vi "Interfaz grafica - corriente.vi"() -> ()   [LabVIEW 2024]
uses:
  160620 Optotune Lens Driver 4 Labview package/Hello Optotune Lens (30.06.2015)/Calibration.ctl
  <vilib>/DAQmx/read.llb/DAQmx Read (Analog 1D Wfm NChan NSamp).vi
  <vilib>/Analysis/2dsp.llb/Decimate (single shot, DBL).vi
  <vilib>/Utility/file.llb/Read Delimited Spreadsheet (string).vi
  <vilib>/Instr/_visa.llb/VISA Configure Serial Port (Instr).vi
  <vilib>/DAQmx/create/channels.llb/DAQmx Create Channel (AI-Voltage-Basic).vi
  <vilib>/DAQmx/configure/timing.llb/DAQmx Timing (Sample Clock).vi
  <vilib>/DAQmx/miscellaneous.llb/DAQmx Fill In Error Info.vi
  <vilib>/Waveform/WDTOps.llb/WDT Index Channel DBL.vi
  <vilib>/Analysis/2dsp.llb/Decimate (continuous, DBL).vi
  <vilib>/Utility/file.llb/Write Delimited Spreadsheet (string).vi
  <vilib>/Waveform/WDTOps.llb/WDT Get Waveform Time Array DBL.vi
  <vilib>/Analysis/NI_AALPro.lvlib
panel:
  out "Array 4":string[](array[string])
  out "Array 3":string[](array[string])
  out "Array 2":string[](array[string])
  out "Array":string[](array[string])
  out "Nombre 2":string
  in  "Restablecer Iniciales":bool
  in  "Incremento":dbl=0.1 format="%#_13g"
  out "Potencia derecho":dbl
  out "error out 4":errorcluster
  out "error out 3":errorcluster
  out "error out 2":errorcluster
  in  "Tab Control 3":enum32{"WL", "Video"}(tab)
  out "Waveform length":dbl[][](graph)
  in  "Minimo escala Y":dbl format="%#_13g"
  in  "Maximo escala Y":dbl format="%#_13g"
  in  "Escala autom. Y":u8=1
  in  "Escala autom. X":u8=1
  in  "Maximo escala X":dbl
  in  "Minimo escala X":dbl
  out "VISA resource name out":string
  in  "Tab Control 2":T1(tab)
  in  "DAQmx Physical Channel":tag
  in  "Frecuencia muestreo":i32=20000
  in  "tamaño buffer":i32=1000
  in  "factor decimacion":i32=20
  in  "Ganancia":u16(ring) items=["0.2"=51455, "1"=33023, "10"=49407, "20"=41215, "30"=57599, "40"=37119, "60"=53503, "80"=45311, "120"=61695, "157"=35071, ""=0]
  in  "Potencia inicial lente derecho":dbl(slide) scale=-3.0..3.0
  in  "Potencia inicial lente izquierdo":dbl(slide) scale=-3.0..3.0
  in  "VISA resource name":string="COM11"
  in  "VISA resource name 2":string="COM10"
  out "DPT INICIALES D":dbl
  out "DPT INICIALES I":dbl
  out "Potencia izquierdo":dbl
  in  "error in (no error) 5":errorcluster
  in  "error in (no error) 4":errorcluster
  in  "error in (no error) 3":errorcluster
  in  "error in (no error) 2":errorcluster
  in  "Calibration 4":T2={"Max Current A"=293.0, "Max Current B"=293.0, "UCL A"=300.0, "UCL B"=300.0, "LCL A"=0.0, "LCL B"=0.0} {"Max Current A" format="%#_g mA"; "Max Current B" format="%#_g mA"; "UCL A" format="%#_g mA"; "LCL A" format="%#_g mA"; "UCL B" format="%#_g mA"; "LCL B" format="%#_g mA"}
  out "ID 2":u16
  out "VISA resource name out 2":string
  out "Calibration 3":T2 {"Max Current A" format="%#_g mA"; "Max Current B" format="%#_g mA"; "UCL A" format="%#_g mA"; "LCL A" format="%#_g mA"; "UCL B" format="%#_g mA"; "LCL B" format="%#_g mA"}
  out "OK 2":bool
  out "Data 2":string
  out "Command to Port 2":string
  in  "Cola tipo 2":dbl[](array[numeric])
  out "Distancia":u32
  in  "Tamaño ventana WL":i32=60
  in  "Limite inferior WL":dbl=25.0 format="%#_13g"
  in  "Limite superior WL":dbl=50.0
  out "number":u32
  in  "Calibration":T2={"Max Current A"=293.0, "Max Current B"=293.0, "UCL A"=300.0, "UCL B"=300.0, "LCL A"=0.0, "LCL B"=0.0} {"Max Current A" format="%#_g mA"; "Max Current B" format="%#_g mA"; "UCL A" format="%#_g mA"; "LCL A" format="%#_g mA"; "UCL B" format="%#_g mA"; "LCL B" format="%#_g mA"}
  out "ID":u16
  out "Calibration 2":T2 {"Max Current A" format="%#_g mA"; "Max Current B" format="%#_g mA"; "UCL A" format="%#_g mA"; "LCL A" format="%#_g mA"; "UCL B" format="%#_g mA"; "LCL B" format="%#_g mA"}
  out "OK":bool
  out "Data":string
  out "Command to Port":string
  in  "DPT dif.":dbl
  out "error out":errorcluster
  in  "error in (no error)":errorcluster
  in  "WL":dbl
  in  "Cola tipo":dbl[](array[numeric])
  out "T button?":bool
  in  "Elegir menu Exp":bool
  in  "Elegir menu":bool
  out "path":path
  in  "Iniciar experimento":bool
  in  "Parar adquisicion":bool
  out "Enfermedad visual":string
  out "Edad":string
  out "Nombre":string
  out "Cedula":string
  in  "Carpeta":path=path "C:/Users/TGM1603/Documents/LabVIEW Data/Experimentos electrodos"
  in  "?":bool
  in  "Menu Principal":u16(ring) items=["Visualizacion general ", "Llevar a cabo un experimento", "Ajustar potencia inicial lentes"]
  in  "Menu experimentos":u16(ring)
  in  "Tab Control":enum32{"Señal EMG", "Potencia y distancia"}(tab)
  out "Senal EMG":waveform(dbl)[](graph)
  in  "Escala automatica Y":u8
  in  "Escala automatica X":u8=1
  in  "X Scale.Range:Increment":dbl
  in  "X Scale.Range:Minimum":dbl
  in  "X Scale.Range:Maximum":dbl
  in  "Y Scale.Range:Minimum":dbl=-5.0
  in  "Y Scale.Range:Maximum":dbl=5.0
  in  "Escala Y min":dbl
  in  "Escala Y max":dbl
  in  "Auto scale Y":u8=1
  in  "Escala X max":dbl
  in  "Escala X min":dbl
  out "Potencia optica y distancia":dbl[][](graph)
  in  "Auto scale X":u8=1
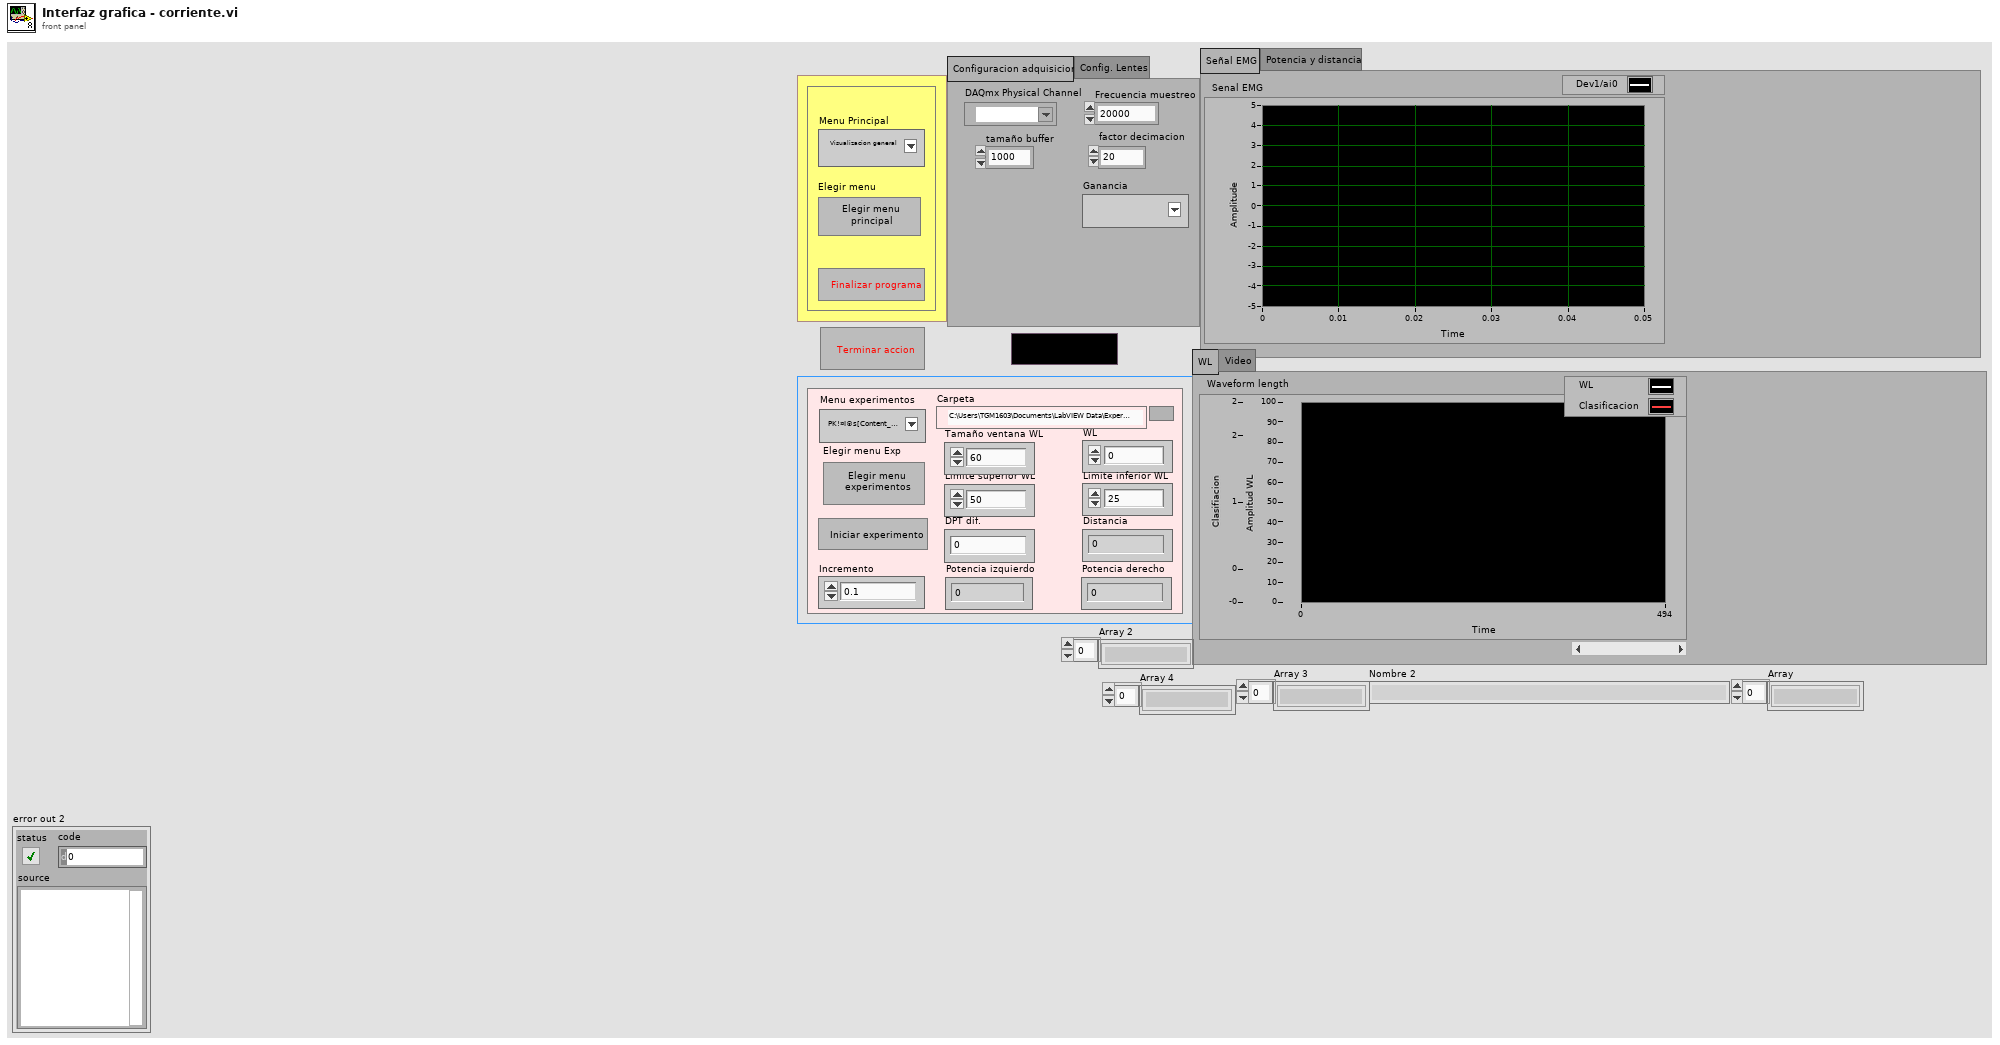
[diagram p1: front panel]
types:
  T1 = enum32{"Configuracion adquisicion", "Config. Lentes"}
  T2 = typedef "Calibration.ctl" = cluster{"Max Current A":dbl, "Max Current B":dbl, "UCL A":dbl, "UCL B":dbl, "LCL A":dbl, "LCL B":dbl}
  T3 = enum16{"Left Button", "Center Button", "Right Button", "Window Close"}
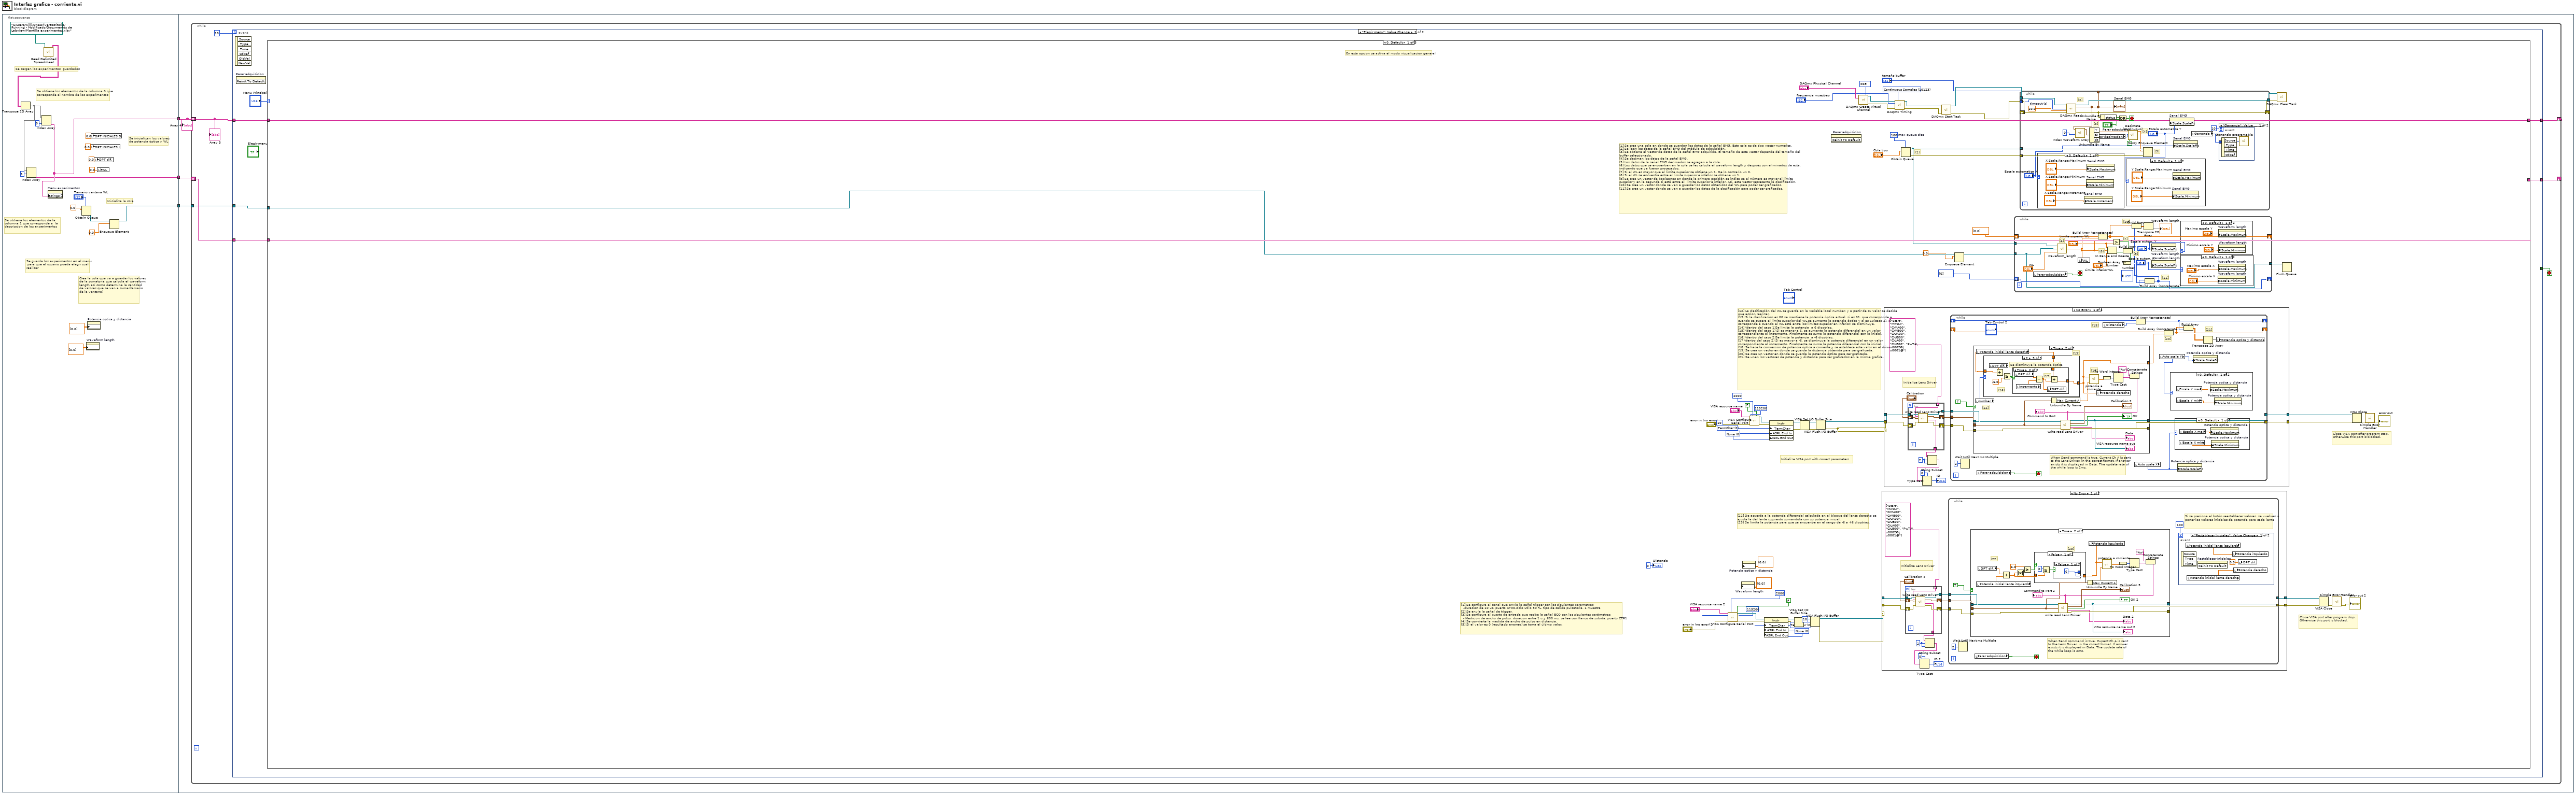
[diagram p0: block diagram]
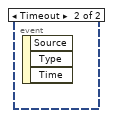
[diagram p2: hidden frame]
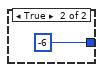
[diagram p4: hidden frame]
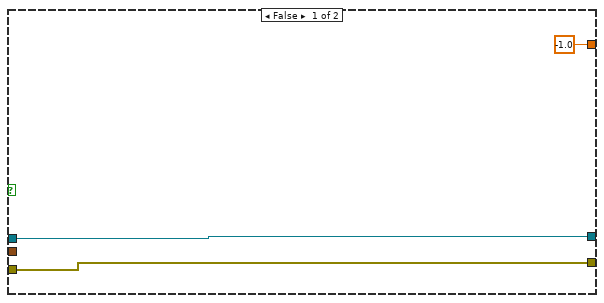
[diagram p9: hidden frame]
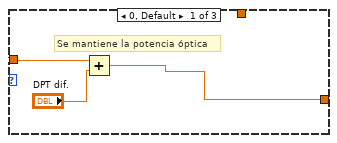
[diagram p10: hidden frame]
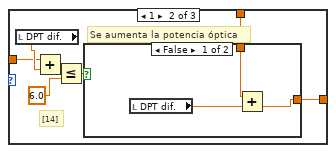
[diagram p11: hidden frame]
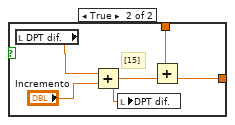
[diagram p12: hidden frame]
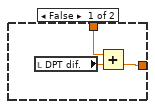
[diagram p13: hidden frame]
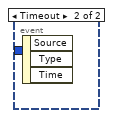
[diagram p17: hidden frame]
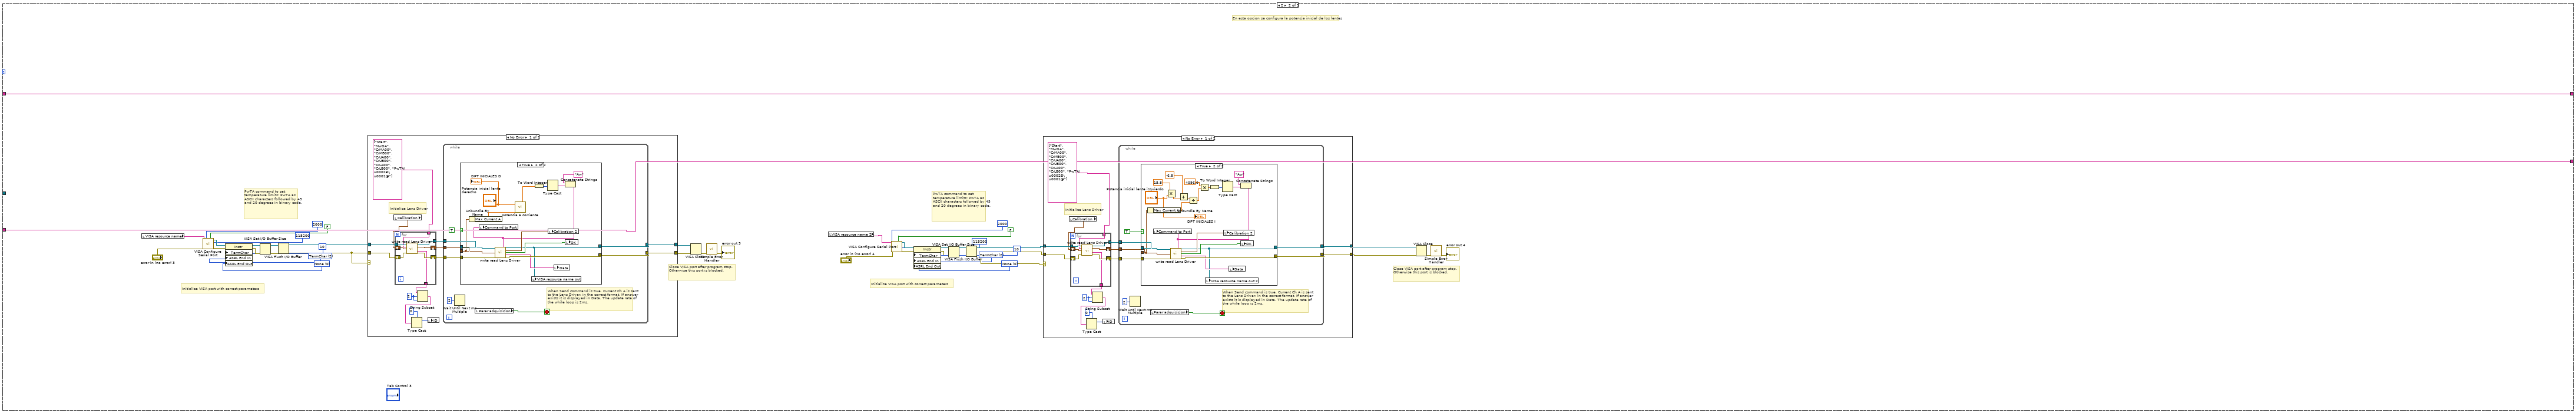
[diagram p20: hidden frame]
diagram:
  n1 = flat-sequence {
    tunnel: [w18] -> w3
    tunnel: [w15] -> w2
    tunnel: [w10] -> w1
    tunnel: w3 -> [w22]
    tunnel: w2 -> [w24]
    tunnel: w1 -> [w23]
    frame #0 {
      # "Se inicializan los valores\nde potencia óptica y WL"
      # "Inicializa la cola"
      # "Crea la cola que va a guardar los valores de la sumatoria que calcula el waveform length así como determina la cantidad de valores que se van a sumar(tamaño de la ventana)"
      # "Se obtiene los elementos de la columna 1 que corresponde a  la descripcion de los experimentos"
      # "Se obtiene los elementos de la columna 0 que corresponde al nombre de los experimentos"
      # "Se guarda los experimentos en el menu\n para que el usuario pueda elegir cual \nrealizar"
      # "Se cargan los experimentos  guardados"
      n2 = call-poly <vilib>:"Read Delimited Spreadsheet.vi"("file path (dialog if empty)"=path "C:/Users/willi/OneDrive/Escritorio/Running - Modificado/Documentos de Labview/Plantilla experimentos.xltx") -> ("all rows"=w19:string[][])  [unwired: 9 in, 5 out]
      n3 = Transpose 2D Array(2D array=w19) -> (transposed array=w16:string[][])
      n4 = Index Array(array=w16, index (row)=1) -> (element=w15:string[])  [unwired: 1 in]
      n5 = Index Array(array=w16, index (row)=0) -> (element=w18:string[])  [unwired: 1 in]
      n6 = property on="Menu experimentos" class="Ring (strict)"("Strings []"=w18) -> ()  [unwired: 2 in, 2 out]
      n7 = Obtain Queue(max queue size (-1, unlimited)="Tamaño ventana WL", element data type=0.0) -> (queue out=w13:refnum<queue>)  [unwired: 3 in, 2 out]
      n8 = property on="Waveform length" class="WFChart (strict)"("History Data"=dbl[][] [[0.0]]) -> ()  [unwired: 2 in, 2 out]
      n9 = property on="Potencia optica y distancia" class="WFChart (strict)"("History Data"=dbl[][] [[0.0]]) -> ()  [unwired: 2 in, 2 out]
      n10 = local write "DPT INICIALES D"(0.0 ("DPT INIT.1")) -> ()
      n11 = local write "DPT INICIALES I"(0.0 ("DPT INIT.2")) -> ()
      n12 = local write "DPT dif."(0.0 ("WL")) -> ()
      n13 = local write "WL"(0.0 ("WL")) -> ()
      n14 = Enqueue Element(queue=w13, element=0.0) -> (queue out=w10:refnum<queue>)  [unwired: 2 in, 2 out]
    }
    frame #1 {
      n15 = while {
        shift-right: [w30] -> _
        shift-left: w22 -> [w31]
        shift-right: [w28] -> _
        shift-left: w24 -> [w29]
        tunnel: w23 -> [w27]
        stop <- w26 stop-if-true
        n16 = event shown="[0] \"Elegir menu\": Value Change" {
          selector: _ -> [_ _]
          dyn-events: _ -> [_ _]
          timeout: 10 -> [_ _]
          tunnel: w31 -> [w37 w1022]
          tunnel: [w36 w1022] -> w30
          tunnel: w29 -> [w35 w1021]
          tunnel: [w34 w1021] -> w28
          tunnel: w27 -> [w32 _]
          tunnel: [_ "?"] -> w26
          event "Elegir menu": Value Change {
            n17 = event-data() -> ()  [unwired: 1 in, 6 out]
            n18 = invoke on="Parar adquisicion" class="Bool (strict)" method="Reinit To Default"() -> ()  [unwired: 3 in, 3 out]
            n19 = case shown="0, Default" "Menu Principal" {
              tunnel: w37 -> [w105 w363 w483]
              tunnel: [w105 w363 w482] -> w36
              tunnel: w35 -> [w104 w362 w480]
              tunnel: [w104 w362 w479] -> w34
              tunnel: w32 -> [w94 _ w470]
              frame 0, Default {
                w39 = 10123 items=["Finite Samples"=10178, "Continuous Samples"=10123, "Hardware Timed Single Point"=12522] ("sample mode")
                w40 = 10083 items=["Default"=-1, "RSE"=10083, "NRSE"=10078, "Differential"=10106, "Pseudodifferential"=12529] ("input terminal configuration")
                w62 = u16 0 items=["None", "Last Bit", "TermChar", "Break"] ("Serial Settings:End Mode for Writes")
                w61 = u16 2 items=["None", "Last Bit", "TermChar"] ("Serial Settings:End Mode for Reads")
                w84 = u16 0 items=["None", "Last Bit", "TermChar", "Break"] ("Serial Settings:End Mode for Writes")
                w85 = u16 2 items=["None", "Last Bit", "TermChar"] ("Serial Settings:End Mode for Reads")
                w98 = 100  # max queue size
                # "[22] De acuerda a la potencia diferencial calculada en el bloque del lente derecho se ajusta la del lente izquierdo sumandola con su potencia inicial.\n[23] Se limita la potencia para que se encuentre en el rango de -6 a +6 dioptrías."
                # "[12] La clasificación del WL se guarda en la variable local number, y a partir de su valor se decide que accion realizar.\n[13] Si la clasificacion es 00 se mantiene la potencia óptica actual, si es 01, que corresponde a cuando se supera el limite superior del WL,se aumenta la potencia óptica y si es 10(caso 2), que corresponde a cuando el WL está entre los limites superior en inferior, se disminuye. \n[14] (dentro del caso 1)Se limita la potencia  a 6 dioptrías. \n[15] (dentro del caso 1) Si es menor a 6, se aumenta la potencia diferencial en un valor correspondiente al incremento. Finalmente se suma la potencia diferencial con la inicial.\n[16] (dentro del caso 2)Se limita la potencia  a -6 dioptrías.\n[17 (dentro del caso 2) Si es mayor a -6, se disminuye la potencia diferencial en un valor correspondiente al incremento. Finalmente se suma la potencia diferencial con la inicial.\n[18] Se hace la conversión de potencia óptica a corriente y se establece este valor en el driver.\n[19] Se crea un vector en donde se guarda la distancia obtenida para ser graficada.\n[20] Se crea un vector en donde se guarda la potencia óptica para ser graficada.\n[21] Se unen los vectores de potencia y distancia para ser graficados en la misma grafica."
                # "[1] Se crea una cola en donde se guardan los datos de la señal EMG. Esta cola es de tipo vector numerica.\n[2] Se leen los datos de la señal EMG del módulo de adquisición. \n[3] Se obtiene el vector de datos de la señal EMG adquirida. El tamaño de este vector depende del tamaño del buffer seleccionado.\n[4] Se deciman los datos de la señal EMG.\n[5] Los datos de la señal EMG decimados se agregan a la cola.\n[6] Los datos que se encuentran en la cola se les calcula el waveform length y después son eliminados de esta, indicando que ya fueron procesados. \n[7] Si el WL es mayor que el limite superior se obtiene un 1. De lo contrario un 0.\n[8] Si el WL se encuentra entre el límite superior e infefior se obtiene un 1.\n[9] Se crea un vector de booleanos en donde la primera posición se indica se el número es mayor al límite superior y en la segunda si está entre el  limite superior e inferior. Así, este vector representa la clasificación.\n[10] Se crea un vector donde se van a guardar los datos obtenidos del WL para poder ser graficados.\n[11] Se crea un vector donde se van a guardar los datos de la clasificación para poder ser graficados."
                # "[1]"
                # "En esta opcion se activa el modo visualizacion general"
                # "Close VISA port after program stop. Otherwise this port is blocked."
                # "[1] Se configura el canal que envía la señal trigger con los siguientes parametros:\n  -duracion de 10 us, puerto CTR0,ciclo utilo 50 %, tipo de salida pulsatoria, 1 muestra \n[2] Se envía la señal de trigger.\n[3] Se configura el puerto de entrada que recibe la señal ECO con los siguientes parámetros:\n  - Medicion de ancho de pulso, duracion entre 1 u y 600 ms, se lee con flanco de subida, puerto CTR1\n[4] Se convierte la medida de ancho de pulso en distancia.\n[5] Si el valor es 0 (resultado erroneo) se toma el último valor."
                # "Close VISA port after program stop. Otherwise this port is blocked."
                # "Initialize VISA port with correct parameters"
                n20 = call-poly "VISA Configure Serial Port"("VISA resource name"="VISA resource name 2", "timeout (10sec)"=u32 2000, "Enable Termination\nChar (T)"=FALSE ("Enable Termination\nChar (T)"), "baud rate (9600)"=u32 115200, "error in (no error)"="error in (no error) 2") -> ("VISA resource name out"=w57:refnum<visa-resource-name>, "error out"=w59:errorcluster)  [unwired: 9 in]
                n21 = property on="Waveform length" class="WFChart (strict)"("History Data"=dbl[][] [[0.0]]) -> ()  [unwired: 2 in, 2 out]
                n22 = property on="Potencia optica y distancia" class="WFChart (strict)"("History Data"=dbl[][] [[0.0]]) -> ()  [unwired: 2 in, 2 out]
                n23 = call-poly "VISA Configure Serial Port"("VISA resource name"="VISA resource name", "timeout (10sec)"=u32 2000, "Enable Termination\nChar (T)"=FALSE ("Enable Termination\nChar (T)"), "baud rate (9600)"=u32 115200, "error in (no error)"="error in (no error)") -> ("VISA resource name out"=w89:refnum<visa-resource-name>, "error out"=w87:errorcluster)  [unwired: 9 in]
                n24 = property class="Instr"(reference=w57, error in=w59, "TermChar"=u8 10 ("Message Based Settings:Termination Character"), "ASRL End In"=w61, "ASRL End Out"=w62) -> (reference out=w58:refnum<visa-resource-name>, error out=w60:errorcluster)
                n25 = property class="Instr"(reference=w89, error in=w87, "TermChar"=u8 10 ("Message Based Settings:Termination Character"), "ASRL End In"=w85, "ASRL End Out"=w84) -> (reference out=w88:refnum<visa-resource-name>, error out=w86:errorcluster)
                n26 = VISA Set I/O Buffer Size(VISA resource name=w58, error in (no error)=w60) -> (VISA resource name out=w65:refnum<visa-resource-name>, error out=w66:errorcluster)  [unwired: 2 in]
                n27 = VISA Set I/O Buffer Size(VISA resource name=w88, error in (no error)=w86) -> (VISA resource name out=w81:refnum<visa-resource-name>, error out=w80:errorcluster)  [unwired: 2 in]
                n28 = VISA Flush I/O Buffer(VISA resource name=w65, error in (no error)=w66) -> (VISA resource name out=w51:refnum<visa-resource-name>, error out=w52:errorcluster)  [unwired: 1 in]
                n29 = VISA Flush I/O Buffer(VISA resource name=w81, error in (no error)=w80) -> (VISA resource name out=w79:refnum<visa-resource-name>, error out=w74:errorcluster)  [unwired: 1 in]
                n30 = invoke on="Parar adquisicion" class="Bool (strict)" method="Reinit To Default"() -> ()  [unwired: 3 in, 3 out]
                n31 = call-poly <vilib>:"DAQmx Create Virtual Channel.vi"("input terminal configuration"=w40, "physical channels"="DAQmx Physical Channel") -> ("task out"=w46:refnum<k21>, "error out"=w45:errorcluster)  [unwired: 12 in]
                n32 = case shown="No Error" w52 {
                  tunnel: w52 -> [w119 w170]
                  tunnel: w51 -> [w118 w171]
                  tunnel: [w117 w170] -> w47
                  tunnel: [w116 w171] -> w48
                  frame No Error {
                    w114 = 2 ("length (rest)")
                    # "Initialize Lens Driver"
                    n33 = for {
                      tunnel: w118 -> [w168]
                      tunnel: [w165] -> w108
                      tunnel: string[] ["Start", "MwDA", "CrMA00", "CrMB00", "CrUA00", "CrUB00", "CrLA00", "CrLB00", "PwTA\u0002Ð\u0001@"] -> [w163] mode=indexing
                      tunnel: [w162] -> w107
                      shift-right: [w166] -> w109
                      shift-left: "Calibration 4" -> [w167]
                      shift-right: [w164] -> w110
                      shift-left: w119 -> [w169]
                      n34 = call "write read Lens Driver.vi"("VISA resource name"=w168, "command"=w163, "Calibration"=w167, "error in (no error)"=w169) -> ("VISA resource name out"=w165:refnum<visa-resource-name>, "Calibration 2"=w166:T2, "Data"=w162:string, "error out"=w164:errorcluster)  [unwired: 4 in, 4 out]
                    }
                    n35 = String Subset(string=w107, offset (0)=w114, length (rest)=w114) -> (substring=w112:string)
                    n36 = Type Cast(type=u16 0 ("length (rest)"), x=w112) -> (*(type *) &x=→"ID 2":u16)
                    n37 = while {
                      tunnel: [w122] -> w117
                      tunnel: [w123] -> w116
                      tunnel: w110 -> [w128]
                      tunnel: w109 -> [w127]
                      tunnel: w108 -> [w126]
                      stop <- w121 stop-if-true
                      # "Si se presiona el botón reestablecer valores, se vuelven a poner los valores iniciales de potencia para cada lente"
                      # "When Send command is true, Current Ch A is sent to the Lens Driver, in the correct format. If answer exists it is displayed in Data. The update rate of the while loop is 2ms."
                      n38 = Wait Until Next ms Multiple(millisecond multiple=u32 2) -> ()  [unwired: 1 out]
                      n39 = case shown="True" TRUE ("Send command") {
                        tunnel: [w133 w154] -> w122
                        tunnel: w128 -> [w133 w153]
                        tunnel: w127 -> [_ w135]
                        tunnel: w126 -> [w132 w152]
                        tunnel: [w132 w149] -> w123
                        frame False {
                        }
                        frame True {
                          # "[23]"
                          # "[22]"
                          n40 = local read "Potencia inicial lente izquierdo"() -> (w143:dbl)
                          n41 = local read "DPT dif."() -> (w144:dbl)
                          n42 = Add(x=w144, y=w143) -> (x+y=w139:dbl)
                          n43 = Absolute Value(x=w139) -> (abs(x)=w141:dbl)
                          n44 = Greater Or Equal?(x=6.0, y=w141) -> (x >= y?=w142:bool)
                          n45 = case shown="False" w142 {
                            tunnel: w139 -> [w157 w161]
                            tunnel: [w155 w161] -> w137
                            frame False {
                              n46 = Greater Or Equal?(x=u16 0, y=w157) -> (x >= y?=w158:bool)
                              n47 = case shown="False" w158 {
                                tunnel: [i16 6 ("x") i16 -6 ("x")] -> w155
                                frame False {
                                }
                                frame True {
                                }
                              }
                            }
                            frame True {
                            }
                          }
                          n48 = Unbundle By Name(w135) -> ("Max Current A"=w136:dbl)
                          n49 = local write "Potencia izquierdo"(w137) -> ()
                          n50 = call "potencia a corriente.vi"("Max current A"=w136, "Potencia"=w137) -> ("Corriente"=w138:dbl)
                          n51 = To Word Integer(number=w138) -> (16bit integer=w147:i16)
                          n52 = Type Cast(x=w147) -> (*(type *) &x=w146:string)  [unwired: 1 in]
                          n53 = Concatenate Strings("Aw", w146) -> (w145:string)
                          "Command to Port 2" <- w145
                          n54 = call "write read Lens Driver.vi"("VISA resource name"=w152, "command"=w145, "Calibration"=w135, "error in (no error)"=w153) -> ("VISA resource name out"=w149:refnum<visa-resource-name>, "Calibration 2"=→"Calibration 3":T2, "OK"=→"OK 2":bool, "Data"=→"Data 2":string, "error out"=w154:errorcluster)  [unwired: 4 in, 3 out]
                          "VISA resource name out 2" <- w149
                        }
                      }
                      n55 = local read "Parar adquisicion"() -> (w121:bool)
                      n56 = event shown="[0] \"Restablecer Iniciales\": Value Change" {
                        selector: _ -> [_ _]
                        dyn-events: _ -> [_ _]
                        timeout: 100 -> [_ _]
                        event "Restablecer Iniciales": Value Change {
                          n57 = event-data() -> ()  [unwired: 1 in, 3 out]
                          n58 = local read "Potencia inicial lente izquierdo"() -> (w129:dbl)
                          n59 = local read "Potencia inicial lente derecho"() -> (w130:dbl)
                          n60 = invoke on="Restablecer Iniciales" class="Bool" method="Reinit To Default"() -> ()  [unwired: 3 in, 3 out]
                          n61 = local write "Potencia izquierdo"(w129) -> ()
                          n62 = local write "Potencia derecho"(w130) -> ()
                          n63 = local write "DPT dif."(0.0 ("DPT dif.")) -> ()
                        }
                        event Timeout {
                          n64 = event-data() -> ()  [unwired: 1 in, 3 out]
                        }
                      }
                    }
                  }
                  frame Error {
                  }
                }
                n65 = case shown="No Error" w74 {
                  tunnel: w74 -> [w185 w269]
                  tunnel: w79 -> [w184 w270]
                  tunnel: [w183 w269] -> w77
                  tunnel: [w182 w270] -> w75
                  frame No Error {
                    w180 = 2 ("length (rest)")
                    # "Initialize Lens Driver"
                    n66 = for {
                      tunnel: w184 -> [w267]
                      tunnel: [w264] -> w174
                      tunnel: string[] ["Start", "MwDA", "CrMA00", "CrMB00", "CrUA00", "CrUB00", "CrLA00", "CrLB00", "PwTA\u0002Ð\u0001@"] -> [w262] mode=indexing
                      tunnel: [w261] -> w173
                      shift-right: [w265] -> w175
                      shift-left: "Calibration" -> [w266]
                      shift-right: [w263] -> w176
                      shift-left: w185 -> [w268]
                      n67 = call "write read Lens Driver.vi"("VISA resource name"=w267, "command"=w262, "Calibration"=w266, "error in (no error)"=w268) -> ("VISA resource name out"=w264:refnum<visa-resource-name>, "Calibration 2"=w265:T2, "Data"=w261:string, "error out"=w263:errorcluster)  [unwired: 4 in, 4 out]
                    }
                    n68 = String Subset(string=w173, offset (0)=w180, length (rest)=w180) -> (substring=w178:string)
                    n69 = Type Cast(type=u16 0 ("length (rest)"), x=w178) -> (*(type *) &x=→"ID":u16)
                    n70 = while {
                      tunnel: [w197] -> w183
                      tunnel: [w198] -> w182
                      tunnel: w176 -> [w203]
                      tunnel: w175 -> [w202]
                      tunnel: w174 -> [w201]
                      shift-right: [w188] -> _
                      shift-left: _ -> [w192]
                      shift-right: [w189] -> _
                      shift-left: _ -> [w191]
                      stop <- w196 stop-if-true
                      # "[21]"
                      # "[20]"
                      # "[19]"
                      # "When Send command is true, Current Ch A is sent to the Lens Driver, in the correct format. If answer exists it is displayed in Data. The update rate of the while loop is 2ms."
                      n71 = Wait Until Next ms Multiple(millisecond multiple=u32 2) -> ()  [unwired: 1 out]
                      n72 = case shown="True" TRUE ("Send command") {
                        tunnel: [w210 w227] -> w197
                        tunnel: w203 -> [w210 w226]
                        tunnel: w202 -> [_ w213]
                        tunnel: w201 -> [w209 w225]
                        tunnel: [w209 w222] -> w198
                        tunnel: [-1.0 ("DPT") w215] -> w190
                        frame False {
                        }
                        frame True {
                          # "[18]"
                          # "[13]"
                          # "[12]"
                          n73 = local read "number"() -> (w217:u32)
                          n74 = local read "Potencia inicial lente derecho"() -> (w216:dbl)
                          n75 = case shown="2" w217 {
                            tunnel: [w229 w237 w252] -> w215
                            tunnel: w216 -> [w230 w232 w247]
                            tunnel: w216 -> [_ w231 w246]
                            frame 0, Default {
                              # "Se mantiene la potencia óptica"
                              n76 = Add(x=w230, y="DPT dif.") -> (x+y=w229:dbl)
                            }
                            frame 1 {
                              # "[14]"
                              # "Se aumenta la potencia óptica"
                              n77 = local read "DPT dif."() -> (w233:dbl)
                              n78 = Add(x=w232, y=w233) -> (x+y=w234:dbl)
                              n79 = Less Or Equal?(x=w234, y=6.0) -> (x <= y?=w236:bool)
                              n80 = case shown="False" w236 {
                                tunnel: [w239 w242] -> w237
                                tunnel: w231 -> [w238 w241]
                                frame False {
                                n81 = local read "DPT dif."() -> (w240:dbl)
                                n82 = Add(x=w238, y=w240) -> (x+y=w239:dbl)
                                }
                                frame True {
                                # "[15]"
                                n83 = local read "DPT dif."() -> (w243:dbl)
                                n84 = Add(x=w243, y="Incremento") -> (x+y=w244:dbl)
                                n85 = local write "DPT dif."(w244) -> ()
                                n86 = Add(x=w241, y=w244) -> (x+y=w242:dbl)
                                }
                              }
                            }
                            frame 2 {
                              # "[16]"
                              # "Se disminuye la potencia óptica"
                              n87 = local read "DPT dif."() -> (w251:dbl)
                              n88 = Add(x=w251, y=w247) -> (x+y=w248:dbl)
                              n89 = Greater Or Equal?(x=w248, y=-6.0) -> (x >= y?=w249:bool)
                              n90 = case shown="True" w249 {
                                tunnel: [w254 w258] -> w252
                                tunnel: w246 -> [w253 w257]
                                frame False {
                                n91 = local read "DPT dif."() -> (w255:dbl)
                                n92 = Add(x=w253, y=w255) -> (x+y=w254:dbl)
                                }
                                frame True {
                                # "[17]"
                                n93 = local read "DPT dif."() -> (w260:dbl)
                                n94 = local read "Incremento"() -> (w256:dbl)
                                n95 = Subtract(x=w260, y=w256) -> (x-y=w259:dbl)
                                n96 = local write "DPT dif."(w259) -> ()
                                n97 = Add(x=w257, y=w259) -> (x+y=w258:dbl)
                                }
                              }
                            }
                          }
                          n98 = Unbundle By Name(w213) -> ("Max Current A"=w212:dbl)
                          n99 = call "potencia a corriente.vi"("Max current A"=w212, "Potencia"=w215) -> ("Corriente"=w214:dbl)
                          n100 = local write "Potencia derecho"(w215) -> ()
                          n101 = To Word Integer(number=w214) -> (16bit integer=w220:i16)
                          n102 = Type Cast(x=w220) -> (*(type *) &x=w219:string)  [unwired: 1 in]
                          n103 = Concatenate Strings("Aw", w219) -> (w218:string)
                          "Command to Port" <- w218
                          n104 = call "write read Lens Driver.vi"("VISA resource name"=w225, "command"=w218, "Calibration"=w213, "error in (no error)"=w226) -> ("VISA resource name out"=w222:refnum<visa-resource-name>, "Calibration 2"=→"Calibration 2":T2, "OK"=→"OK":bool, "Data"=→"Data":string, "error out"=w227:errorcluster)  [unwired: 4 in, 3 out]
                          "VISA resource name out" <- w222
                        }
                      }
                      n105 = local read "Parar adquisicion"() -> (w196:bool)
                      n106 = local read "Distancia"() -> (w193:u32)
                      n107 = local read "Auto scale X"() -> (w194:u8)
                      n108 = Build Array (concatenate)(w192, w193) -> (w188:u32[])
                      n109 = local read "Auto scale Y"() -> (w195:u8)
                      n110 = Build Array (concatenate)(w191, w190) -> (w189:dbl[])
                      n111 = case shown="0, Default" w195 {
                        frame 0, Default {
                          n112 = local read "Escala Y max"() -> (w207:dbl)
                          n113 = local read "Escala Y min"() -> (w206:dbl)
                          n114 = property on="Potencia optica y distancia" class="WFChart (strict)"("YScale.Maximum"=w207) -> ()  [unwired: 2 in, 2 out]
                          n115 = property on="Potencia optica y distancia" class="WFChart (strict)"("YScale.Minimum"=w206) -> ()  [unwired: 2 in, 2 out]
                        }
                        frame 1 {
                        }
                      }
                      n116 = case shown="0, Default" w194 {
                        frame 0, Default {
                          n117 = local read "Escala X min"() -> (w204:dbl)
                          n118 = local read "Escala X max"() -> (w205:dbl)
                          n119 = property on="Potencia optica y distancia" class="WFChart (strict)"("XScale.Maximum"=w205) -> ()  [unwired: 2 in, 2 out]
                          n120 = property on="Potencia optica y distancia" class="WFChart (strict)"("XScale.Minimum"=w204) -> ()  [unwired: 2 in, 2 out]
                        }
                        frame 1 {
                        }
                      }
                      n121 = property on="Potencia optica y distancia" class="WFChart (strict)"("XScale.ScaleFit"=w194) -> ()  [unwired: 2 in, 2 out]
                      n122 = Build Array(w189, w188) -> (w187:dbl[][])
                      n123 = property on="Potencia optica y distancia" class="WFChart (strict)"("YScale.ScaleFit"=w195) -> ()  [unwired: 2 in, 2 out]
                      n124 = Transpose 2D Array(2D array=w187) -> (transposed array=w186:dbl[][])
                      n125 = local write "Potencia optica y distancia"(w186) -> ()
                    }
                  }
                  frame Error {
                  }
                }
                n126 = call-poly <vilib>:"DAQmx Timing.vi"("task/channels in"=w46, "sample mode"=w39, "rate"="Frecuencia muestreo", "error in"=w45) -> ("task out"=w44:refnum<k21>, "error out"=w43:errorcluster)  [unwired: 10 in]
                n127 = Obtain Queue(max queue size (-1, unlimited)=w98, element data type="Cola tipo") -> (queue out=w95:refnum<queue>, error out=w96:errorcluster)  [unwired: 3 in, 1 out]
                n128 = call <vilib>:"DAQmx Start Task.vi"("task/channels in"=w44, "error in"=w43) -> ("task out"=w103:refnum<k21>, "error out"=w102:errorcluster)  [unwired: 12 in]
                n129 = Enqueue Element(queue=w94, element=0.0) -> (queue out=w71:refnum<queue>)  [unwired: 2 in, 2 out]
                n130 = while {
                  tunnel: w71 -> [w272]
                  tunnel: w95 -> [w289]
                  shift-right: [w275] -> _
                  shift-left: dbl[] [0.0] -> [w286]
                  shift-right: [w274] -> _
                  shift-left: u32[] [0] -> [w276]
                  tunnel: [w272] -> w69
                  stop <- w287 stop-if-true
                  # "[11]"
                  # "[10]"
                  # "[9]"
                  # "[8]"
                  # "[7]"
                  # "[6]"
                  n131 = local read "Parar adquisicion"() -> (w287:bool)
                  n132 = call "waveform_length.vi"("WL"="WL", "Cola WL"=w272, "Datos entrada"=w289) -> ("WL 2"=w284:dbl)
                  n133 = local write "WL"(w284) -> ()
                  n134 = Build Array (concatenate)(w286, w284) -> (w275:dbl[])
                  n135 = In Range and Coerce(upper limit="Limite superior WL", x=w284, lower limit="Limite inferior WL") -> (In Range?=w282:bool)  [unwired: 1 out]
                  n136 = Greater?(x=w284, y="Limite superior WL") -> (0:w283:bool)
                  n137 = Build Array(w283, w282) -> (w281:bool[])
                  n138 = Boolean Array To Number(Boolean array=w281) -> (number=w277:u32)
                  "number" <- w277
                  n139 = Build Array (concatenate)(w276, w277) -> (w274:u32[])
                  n140 = Build Array(w275, w274) -> (w273:dbl[][])
                  n141 = Transpose 2D Array(2D array=w273) -> (transposed array=→"Waveform length":dbl[][])
                  n142 = property on="Waveform length" class="WFChart (strict)"("YScale.ScaleFit"="Escala autom. Y") -> ()  [unwired: 2 in, 2 out]
                  n143 = property on="Waveform length" class="WFChart (strict)"("XScale.ScaleFit"="Escala autom. X") -> ()  [unwired: 2 in, 2 out]
                  n144 = case shown="0, Default" "Escala autom. Y" {
                    frame 0, Default {
                      n145 = property on="Waveform length" class="WFChart (strict)"("YScale.Maximum"="Maximo escala Y") -> ()  [unwired: 2 in, 2 out]
                      n146 = property on="Waveform length" class="WFChart (strict)"("YScale.Minimum"="Minimo escala Y") -> ()  [unwired: 2 in, 2 out]
                    }
                    frame 1 {
                    }
                  }
                  n147 = case shown="0, Default" "Escala autom. X" {
                    frame 0, Default {
                      n148 = property on="Waveform length" class="WFChart (strict)"("XScale.Minimum"="Minimo escala X") -> ()  [unwired: 2 in, 2 out]
                      n149 = property on="Waveform length" class="WFChart (strict)"("XScale.Maximum"="Maximo escala X") -> ()  [unwired: 2 in, 2 out]
                    }
                    frame 1 {
                    }
                  }
                }
                n150 = while {
                  tunnel: w103 -> [w315]
                  tunnel: "tamaño buffer" -> [w312]
                  tunnel: [w313] -> w99
                  shift-right: [w310] -> w100
                  shift-left: w102 -> [w314]
                  tunnel: [w304] -> _
                  tunnel: w95 -> [w300]
                  tunnel: w96 -> [w299]
                  stop <- w309 stop-if-true
                  w308 = 10.0  # timeout (s)
                  # "[5]"
                  # "[4]"
                  # "[3]"
                  # "[2]"
                  n151 = case shown="0, Default" "Escala automatica X" {
                    frame 0, Default {
                      n152 = property on="Senal EMG" class="WFGraph (strict)"("XScale.Increment"="X Scale.Range:Increment") -> ()  [unwired: 2 in, 2 out]
                      n153 = property on="Senal EMG" class="WFGraph (strict)"("XScale.Minimum"="X Scale.Range:Minimum") -> ()  [unwired: 2 in, 2 out]
                      n154 = property on="Senal EMG" class="WFGraph (strict)"("XScale.Maximum"="X Scale.Range:Maximum") -> ()  [unwired: 2 in, 2 out]
                    }
                    frame 1 {
                    }
                  }
                  n155 = call-poly <vilib>:"DAQmx Read.vi"("task/channels in"=w315, "number of samples per channel"=w312, "timeout"=w308, "error in"=w314) -> ("task out"=w313:refnum<k21>, "data"=w304:waveform(dbl)[], "error out"=w310:errorcluster)  [unwired: 9 in]
                  "Senal EMG" <- w304
                  n156 = call-poly <vilib>:"Index Waveform Array.vi"("index"=0, "waveform array"=w304) -> ("waveform"=w305:waveform(dbl))  [unwired: 8 in, 1 out]
                  n157 = Unbundle By Name(w305) -> ("Y"=w302:dbl[])  [unwired: 2 out]
                  n158 = local read "factor decimacion"() -> (w301:i32)
                  n159 = Unbundle By Name(w310) -> ("status"=w311:bool)
                  n160 = Or(x=w311, y="Parar adquisicion") -> (x .or. y?=w309:bool)
                  n161 = case shown="0, Default" "Escala automatica Y" {
                    frame 0, Default {
                      n162 = property on="Senal EMG" class="WFGraph (strict)"("YScale.Minimum"="Y Scale.Range:Minimum") -> ()  [unwired: 2 in, 2 out]
                      n163 = property on="Senal EMG" class="WFGraph (strict)"("YScale.Maximum"="Y Scale.Range:Maximum") -> ()  [unwired: 2 in, 2 out]
                    }
                    frame 1 {
                    }
                  }
                  n164 = call-poly <vilib>:"Decimate (continuous).vi"("averaging"=TRUE, "decimating factor"=w301, "X"=w302) -> ("Decimated Array"=w298:dbl[])  [unwired: 7 in, 1 out]
                  n165 = Lossy Enqueue Element(queue=w300, element=w298, error in (no error)=w299) -> ()  [unwired: 4 out]
                  n166 = property on="Senal EMG" class="WFGraph (strict)"("YScale.ScaleFit"="Escala automatica Y") -> ()  [unwired: 2 in, 2 out]
                  n167 = property on="Senal EMG" class="WFGraph (strict)"("XScale.ScaleFit"="Escala automatica X") -> ()  [unwired: 2 in, 2 out]
                  n168 = local read "Ganancia"() -> (w295:u16)
                  n169 = event shown="[0] \"Ganancia\": Value Change" {
                    selector: _ -> [_ _]
                    dyn-events: _ -> [_ _]
                    timeout: 10 -> [_ _]
                    tunnel: w295 -> [w316 _]
                    event "Ganancia": Value Change {
                      n170 = event-data() -> ()  [unwired: 1 in, 4 out]
                      n171 = call "Ganancia programable.vi"("MOSI data"=w316) -> ()
                    }
                    event Timeout {
                      n172 = event-data() -> ()  [unwired: 1 in, 3 out]
                    }
                  }
                }
                n173 = call <vilib>:"DAQmx Clear Task.vi"("task in"=w99, "error in"=w100) -> ()  [unwired: 13 in, 1 out]
                n174 = Flush Queue(queue=w69) -> ()  [unwired: 1 in, 3 out]
                n175 = VISA Close(VISA resource name=w48, error in (no error)=w47) -> (error out=w49:errorcluster)
                n176 = call <vilib>:"Simple Error Handler.vi"("error in (no error)"=w49) -> ("error out"=→"error out 2":errorcluster)  [unwired: 4 in, 4 out]
                n177 = VISA Close(VISA resource name=w75, error in (no error)=w77) -> (error out=w78:errorcluster)
                n178 = call <vilib>:"Simple Error Handler.vi"("error in (no error)"=w78) -> ("error out"=→"error out":errorcluster)  [unwired: 4 in, 4 out]
                "Distancia" <- u32 0 ("Distancia")
              }
              frame 2 {
                w342 = u16 0 items=["None", "Last Bit", "TermChar", "Break"] ("Serial Settings:End Mode for Writes")
                w341 = u16 2 items=["None", "Last Bit", "TermChar"] ("Serial Settings:End Mode for Reads")
                w355 = u16 0 items=["None", "Last Bit", "TermChar", "Break"] ("Serial Settings:End Mode for Writes")
                w354 = u16 2 items=["None", "Last Bit", "TermChar"] ("Serial Settings:End Mode for Reads")
                # "En esta opcion se configura la potencia inicial de los lentes"
                # "Close VISA port after program stop. Otherwise this port is blocked."
                # "Close VISA port after program stop. Otherwise this port is blocked."
                # "PwTA command to set temperature limits: PwTA as ASCII characters followed by 45 and 20 degrees in binary code."
                # "Initialize VISA port with correct parameters"
                # "PwTA command to set temperature limits: PwTA as ASCII characters followed by 45 and 20 degrees in binary code."
                # "Initialize VISA port with correct parameters"
                n179 = local read "VISA resource name"() -> (w332:string)
                n180 = call-poly "VISA Configure Serial Port"("VISA resource name"=w332, "timeout (10sec)"=u32 2000, "Enable Termination\nChar (T)"=FALSE ("Enable Termination\nChar (T)"), "baud rate (9600)"=u32 115200, "error in (no error)"="error in (no error) 3") -> ("VISA resource name out"=w337:refnum<visa-resource-name>, "error out"=w339:errorcluster)  [unwired: 9 in]
                n181 = property class="Instr"(reference=w337, error in=w339, "TermChar"=u8 10 ("Message Based Settings:Termination Character"), "ASRL End In"=w341, "ASRL End Out"=w342) -> (reference out=w338:refnum<visa-resource-name>, error out=w340:errorcluster)
                n182 = VISA Set I/O Buffer Size(VISA resource name=w338, error in (no error)=w340) -> (VISA resource name out=w344:refnum<visa-resource-name>, error out=w345:errorcluster)  [unwired: 2 in]
                n183 = VISA Flush I/O Buffer(VISA resource name=w344, error in (no error)=w345) -> (VISA resource name out=w331:refnum<visa-resource-name>, error out=w330:errorcluster)  [unwired: 1 in]
                n184 = case shown="No Error" w330 {
                  tunnel: w330 -> [w377 w411]
                  tunnel: w331 -> [w376 w412]
                  tunnel: [w375 w411] -> w326
                  tunnel: [w374 w412] -> w327
                  frame No Error {
                    w373 = 2 ("length (rest)")
                    # "Initialize Lens Driver"
                    n185 = local read "Calibration"() -> (w365:T2)
                    n186 = for {
                      tunnel: w376 -> [w409]
                      tunnel: [w406] -> w368
                      tunnel: string[] ["Start", "MwDA", "CrMA00", "CrMB00", "CrUA00", "CrUB00", "CrLA00", "CrLB00", "PwTA\u0002Ð\u0001@"] -> [w404] mode=indexing
                      tunnel: [w403] -> w367
                      shift-right: [w407] -> w369
                      shift-left: w365 -> [w408]
                      shift-right: [w405] -> w370
                      shift-left: w377 -> [w410]
                      n187 = call "write read Lens Driver.vi"("VISA resource name"=w409, "command"=w404, "Calibration"=w408, "error in (no error)"=w410) -> ("VISA resource name out"=w406:refnum<visa-resource-name>, "Calibration 2"=w407:T2, "Data"=w403:string, "error out"=w405:errorcluster)  [unwired: 4 in, 4 out]
                    }
                    n188 = String Subset(string=w367, offset (0)=w373, length (rest)=w373) -> (substring=w371:string)
                    n189 = Type Cast(type=u16 0 ("length (rest)"), x=w371) -> (*(type *) &x=w366:u16)
                    n190 = local write "ID"(w366) -> ()
                    n191 = while {
                      tunnel: [w379] -> w375
                      tunnel: [w380] -> w374
                      tunnel: w370 -> [w385]
                      tunnel: w369 -> [w384]
                      tunnel: w368 -> [w383]
                      stop <- w378 stop-if-true
                      # "When Send command is true, Current Ch A is sent to the Lens Driver, in the correct format. If answer exists it is displayed in Data. The update rate of the while loop is 2ms."
                      n192 = Wait Until Next ms Multiple(millisecond multiple=u32 2) -> ()  [unwired: 1 out]
                      n193 = case shown="True" TRUE ("Send command") {
                        tunnel: [w387 w402] -> w379
                        tunnel: w385 -> [w387 w401]
                        tunnel: w384 -> [_ w392]
                        tunnel: w383 -> [w386 w400]
                        tunnel: [w386 w393] -> w380
                        frame False {
                        }
                        frame True {
                          n194 = Unbundle By Name(w392) -> ("Max Current A"=w391:dbl)
                          n195 = call "potencia a corriente.vi"("Max current A"=w391, "Potencia"="Potencia inicial lente derecho") -> ("Corriente"=w389:dbl)
                          n196 = To Word Integer(number=w389) -> (16bit integer=w399:i16)
                          n197 = Type Cast(x=w399) -> (*(type *) &x=w398:string)  [unwired: 1 in]
                          n198 = Concatenate Strings("Aw", w398) -> (w395:string)
                          n199 = local write "Command to Port"(w395) -> ()
                          n200 = call "write read Lens Driver.vi"("VISA resource name"=w400, "command"=w395, "Calibration"=w392, "error in (no error)"=w401) -> ("VISA resource name out"=w393:refnum<visa-resource-name>, "Calibration 2"=w397:T2, "OK"=w396:bool, "Data"=w394:string, "error out"=w402:errorcluster)  [unwired: 4 in, 3 out]
                          n201 = local write "VISA resource name out"(w393) -> ()
                          n202 = local write "Calibration 2"(w397) -> ()
                          n203 = local write "Data"(w394) -> ()
                          n204 = local write "OK"(w396) -> ()
                          "DPT INICIALES D" <- "Potencia inicial lente derecho"
                        }
                      }
                      n205 = local read "Parar adquisicion"() -> (w378:bool)
                    }
                  }
                  frame Error {
                  }
                }
                n206 = VISA Close(VISA resource name=w327, error in (no error)=w326) -> (error out=w329:errorcluster)
                n207 = call <vilib>:"Simple Error Handler.vi"("error in (no error)"=w329) -> ("error out"=→"error out 3":errorcluster)  [unwired: 4 in, 4 out]
                n208 = local read "VISA resource name 2"() -> (w346:string)
                n209 = call-poly "VISA Configure Serial Port"("VISA resource name"=w346, "timeout (10sec)"=u32 2000, "Enable Termination\nChar (T)"=FALSE ("Enable Termination\nChar (T)"), "baud rate (9600)"=u32 115200, "error in (no error)"="error in (no error) 4") -> ("VISA resource name out"=w350:refnum<visa-resource-name>, "error out"=w352:errorcluster)  [unwired: 9 in]
                n210 = property class="Instr"(reference=w350, error in=w352, "TermChar"=u8 10 ("Message Based Settings:Termination Character"), "ASRL End In"=w354, "ASRL End Out"=w355) -> (reference out=w351:refnum<visa-resource-name>, error out=w353:errorcluster)
                n211 = VISA Set I/O Buffer Size(VISA resource name=w351, error in (no error)=w353) -> (VISA resource name out=w357:refnum<visa-resource-name>, error out=w358:errorcluster)  [unwired: 2 in]
                n212 = VISA Flush I/O Buffer(VISA resource name=w357, error in (no error)=w358) -> (VISA resource name out=w360:refnum<visa-resource-name>, error out=w359:errorcluster)  [unwired: 1 in]
                n213 = case shown="No Error" w359 {
                  tunnel: w359 -> [w426 w466]
                  tunnel: w360 -> [w425 w467]
                  tunnel: [w424 w466] -> w323
                  tunnel: [w423 w467] -> w322
                  frame No Error {
                    w422 = 2 ("length (rest)")
                    # "Initialize Lens Driver"
                    n214 = local read "Calibration"() -> (w414:T2)
                    n215 = for {
                      tunnel: w425 -> [w464]
                      tunnel: [w461] -> w417
                      tunnel: string[] ["Start", "MwDA", "CrMA00", "CrMB00", "CrUA00", "CrUB00", "CrLA00", "CrLB00", "PwTA\u0002Ð\u0001@"] -> [w459] mode=indexing
                      tunnel: [w458] -> w416
                      shift-right: [w462] -> w418
                      shift-left: w414 -> [w463]
                      shift-right: [w460] -> w419
                      shift-left: w426 -> [w465]
                      n216 = call "write read Lens Driver.vi"("VISA resource name"=w464, "command"=w459, "Calibration"=w463, "error in (no error)"=w465) -> ("VISA resource name out"=w461:refnum<visa-resource-name>, "Calibration 2"=w462:T2, "Data"=w458:string, "error out"=w460:errorcluster)  [unwired: 4 in, 4 out]
                    }
                    n217 = String Subset(string=w416, offset (0)=w422, length (rest)=w422) -> (substring=w420:string)
                    n218 = Type Cast(type=u16 0 ("length (rest)"), x=w420) -> (*(type *) &x=w415:u16)
                    n219 = local write "ID"(w415) -> ()
                    n220 = while {
                      tunnel: [w428] -> w424
                      tunnel: [w429] -> w423
                      tunnel: w419 -> [w434]
                      tunnel: w418 -> [w433]
                      tunnel: w417 -> [w432]
                      stop <- w427 stop-if-true
                      # "When Send command is true, Current Ch A is sent to the Lens Driver, in the correct format. If answer exists it is displayed in Data. The update rate of the while loop is 2ms."
                      n221 = Wait Until Next ms Multiple(millisecond multiple=u32 2) -> ()  [unwired: 1 out]
                      n222 = case shown="True" TRUE ("Send command") {
                        tunnel: [w436 w457] -> w428
                        tunnel: w434 -> [w436 w456]
                        tunnel: w433 -> [_ w444]
                        tunnel: w432 -> [w435 w455]
                        tunnel: [w435 w445] -> w429
                        frame False {
                        }
                        frame True {
                          n223 = Unbundle By Name(w444) -> ("Max Current A"=w443:dbl)
                          n224 = Multiply(x=15.8, y="Potencia inicial lente izquierdo") -> (x*y=w441:dbl)
                          n225 = Add(x=-6.8, y=w441) -> (x+y=w439:dbl)
                          n226 = Divide(x=w439, y=w443) -> (x/y=w442:dbl)
                          n227 = Multiply(x=4096.0, y=w442) -> (x*y=w453:dbl)
                          n228 = To Word Integer(number=w453) -> (16bit integer=w452:i16)
                          n229 = Type Cast(x=w452) -> (*(type *) &x=w451:string)  [unwired: 1 in]
                          n230 = Concatenate Strings("Aw", w451) -> (w447:string)
                          n231 = local write "Command to Port"(w447) -> ()
                          n232 = call "write read Lens Driver.vi"("VISA resource name"=w455, "command"=w447, "Calibration"=w444, "error in (no error)"=w456) -> ("VISA resource name out"=w445:refnum<visa-resource-name>, "Calibration 2"=w449:T2, "OK"=w448:bool, "Data"=w446:string, "error out"=w457:errorcluster)  [unwired: 4 in, 3 out]
                          n233 = local write "VISA resource name out 2"(w445) -> ()
                          n234 = local write "Calibration 2"(w449) -> ()
                          n235 = local write "Data"(w446) -> ()
                          n236 = local write "OK"(w448) -> ()
                          "DPT INICIALES I" <- "Potencia inicial lente izquierdo"
                        }
                      }
                      n237 = local read "Parar adquisicion"() -> (w427:bool)
                    }
                  }
                  frame Error {
                  }
                }
                n238 = VISA Close(VISA resource name=w322, error in (no error)=w323) -> (error out=w325:errorcluster)
                n239 = call <vilib>:"Simple Error Handler.vi"("error in (no error)"=w325) -> ("error out"=→"error out 4":errorcluster)  [unwired: 4 in, 4 out]
              }
              frame 1 {
                # "Mensaje que pregunta si desea realizar el experimento\ncon un nuevo usuario o con el actual"
                # "Se vuelven 0 los valores del WL y de la potencia óptica y distancia"
                # "En esta opcion se activa el modo experimento"
                n240 = property on="Waveform length" class="WFChart (strict)"("History Data"=dbl[][] [[0.0]]) -> ()  [unwired: 2 in, 2 out]
                n241 = property on="Potencia optica y distancia" class="WFChart (strict)"("History Data"=dbl[][] [[0.0]]) -> ()  [unwired: 2 in, 2 out]
                n242 = Two Button Dialog(message="Con quien desea realizar los experimentos?", 1:"Nuevo voluntario" ("F button name (\"Cancel\")"), 2:"Voluntario actual" ("T button name (\"OK\")")) -> (T button?=w486:bool)
                n243 = flat-sequence {
                  tunnel: w486 -> [w499]
                  tunnel: [w498] -> w484
                  tunnel: w483 -> [w498]
                  tunnel: [w491] -> w471
                  tunnel: w470 -> [w491]
                  tunnel: [w509] -> w487
                  tunnel: [w511] -> w485
                  tunnel: w484 -> [w511]
                  tunnel: [w510] -> w481
                  tunnel: w480 -> [w510]
                  tunnel: [w508] -> w472
                  tunnel: w471 -> [w508]
                  tunnel: w487 -> [w523]
                  tunnel: w485 -> [w522]
                  tunnel: [w521] -> w482
                  tunnel: w481 -> [w520]
                  tunnel: [w519] -> w478
                  tunnel: [w518] -> w477
                  tunnel: [w517] -> w475
                  tunnel: [w516] -> w473
                  tunnel: w472 -> [w516]
                  tunnel: w478 -> [w575]
                  tunnel: w477 -> [w558]
                  tunnel: [w575] -> w476
                  tunnel: w475 -> [w561]
                  tunnel: [w549] -> w474
                  tunnel: w473 -> [w549]
                  tunnel: [w578] -> w479
                  tunnel: w476 -> [w578]
                  tunnel: w474 -> [w576]
                  frame #0 {
                    # "Se guardan los datos de un nuevo voluntario"
                    n244 = Not(x=w499) -> (.not. x?=w493:bool)
                    n245 = case shown="True" w493 {
                      tunnel: [w502 w507] -> w497
                      tunnel: [w501 w506] -> w496
                      tunnel: [w503 w505] -> w495
                      tunnel: [w500 w504] -> w494
                      frame False {
                        n246 = local read "Enfermedad visual"() -> (w502:string)
                        n247 = local read "Nombre"() -> (w503:string)
                        n248 = local read "Cedula"() -> (w500:string)
                        n249 = local read "Edad"() -> (w501:string)
                      }
                      frame True {
                        n250 = call "Registro voluntario"() -> ("Enfermedad visual"=w507:string, "Edad"=w506:string, "Cedula"=w504:string, "Nombre"=w505:string)  [unwired: 14 in, 2 out]
                      }
                    }
                    "Cedula" <- w494
                    "Nombre" <- w495
                    "Edad" <- w496
                    "Enfermedad visual" <- w497
                    n251 = local write "T button?"(FALSE ("T button?")) -> ()
                  }
                  frame #1 {
                    n252 = Two Button Dialog(message="Qué tipo de experimento desea realizar?", 1:"Nuevo Experimento" ("F button name (\"Cancel\")"), 2:"Experimento existente" ("T button name (\"OK\")")) -> (T button?=w512:bool)
                    n253 = Not(x=w512) -> (.not. x?=w509:bool)
                  }
                  frame #2 {
                    # "A partir de la seleccion del experimento, se obtiene la descripcion correspondiente que será guardada en el archivo"
                    n254 = case shown="False" w523 {
                      tunnel: w522 -> [w525 w543]
                      tunnel: [w525 w542] -> w521
                      tunnel: w520 -> [w527 w541]
                      tunnel: [w527 w540] -> w519
                      tunnel: [w528 w539] -> w518
                      tunnel: [w524 w538] -> w517
                      frame False {
                        n255 = call "Display Message to User"() -> ()  [unwired: 10 in, 2 out]
                        n256 = flat-sequence {
                          tunnel: [w529] -> w526
                          tunnel: w525 -> [w529]
                          tunnel: [w537] -> w528
                          tunnel: w527 -> [w536]
                          tunnel: ["Menu experimentos"] -> _
                          tunnel: w526 -> [w534]
                          tunnel: [w533] -> w524
                          frame #0 {
                            n257 = while {
                              stop <- w530 stop-if-true
                              # "El sistema se queda en el loop hasta que el usuario elija el experimento que desea realizar"
                              n258 = event shown="[0] \"Elegir menu Exp\": Value Change" {
                                selector: _ -> [_ _]
                                dyn-events: _ -> [_ _]
                                timeout: _ -> [_ _]
                                tunnel: [TRUE FALSE] -> w530
                                event "Elegir menu Exp": Value Change {
                                n259 = event-data() -> ()  [unwired: 1 in, 4 out]
                                }
                                event Timeout {
                                n260 = event-data() -> ()  [unwired: 1 in, 3 out]
                                }
                              }
                            }
                          }
                          frame #1 {
                            n261 = Index Array(array=w536, index="Menu experimentos") -> (element=w537:string)
                            n262 = Index Array(array=w534, index="Menu experimentos") -> (element=w533:string)
                          }
                        }
                        "Array" <- w525
                      }
                      frame True {
                        # "Se añade el nuevo experimento al menu de seleccion de experimentos"
                        # "Se guarda el nuevo experimento en el archivo que los contiene"
                        n263 = call "Nuevo experimento"() -> ("Descripcion"=w539:string, "Nombre"=w538:string)  [unwired: 16 in, 2 out]
                        n264 = Insert Into Array(array=w541, new element=w539) -> (w540:string[])  [unwired: 1 in]
                        n265 = Insert Into Array(array=w543, new element=w538) -> (w542:string[])  [unwired: 1 in]
                        n266 = property on="Menu experimentos" class="Ring (strict)"("Strings []"=w542) -> ()  [unwired: 2 in, 2 out]
                        n267 = Insert Into Array(array=string[] [], new element #1=w538, new element #2=w539) -> (w545:string[])  [unwired: 1 in]
                        n268 = call-poly <vilib>:"Write Delimited Spreadsheet.vi"("file path (dialog if empty)"=path "C:/Users/TGM1603/Documents/LabVIEW Data/Experimentos_realizados", "1D data"=w545, "append to file? (new file:F)"=TRUE) -> ()  [unwired: 11 in, 2 out]
                      }
                    }
                  }
                  frame #3 {
                    # "Se guardan los datos generales del experimento en el archivo de excel"
                    n269 = local read "Frecuencia muestreo"() -> (w551:i32)
                    n270 = local read "factor decimacion"() -> (w557:i32)
                    n271 = local read "Enfermedad visual"() -> (w560:string)
                    n272 = local read "Cedula"() -> (w562:string)
                    n273 = local read "Edad"() -> (w559:string)
                    n274 = local read "Nombre"() -> (w563:string)
                    n275 = Get Date/Time In Seconds() -> (seconds since 1Jan1904=w574:timestamp)
                    n276 = Path To String(path="Carpeta") -> (string=w570:string)
                    n277 = Format Date/Time String(time format string (%c)="_%d-%m-%y_%H-%M", seconds (now)=w574) -> (date/time string=w572:string)  [unwired: 1 in]
                    n278 = Number To Fractional String(number=0.0, precision (6)=i16 0) -> (F-format string=w554:string)  [unwired: 2 in]
                    n279 = Number To Fractional String(number=w557, precision (6)=i16 0) -> (F-format string=w556:string)  [unwired: 2 in]
                    n280 = local read "Cedula"() -> (w566:string)
                    n281 = Number To Fractional String(number=w551, precision (6)=i16 0) -> (F-format string=w552:string)  [unwired: 2 in]
                    n282 = Concatenate Strings(w570, "\\" ("string"), w566, w572, "_" ("string"), w561, ".xlsx" ("string")) -> (w568:string)
                    n283 = String To Path(string=w568) -> (path=w567:path)
                    "path" <- w567
                    n284 = call "MS Office Report"("Path to Save Report"=w567, "Cedula"=w562, "decimacion"=w556, "Edad"=w559, "Enfermedad"=w560, "Exp_nombre"=w561, "Experimento"=w558, "freq"=w552, "Nombre"=w563, "rango"=w554) -> ()  [unwired: 16 in, 2 out]
                    "Nombre 2" <- w561
                  }
                  frame #4 {
                    n285 = while {
                      shift-right: [w580] -> _
                      shift-left: enum16{"Inicio", "Tomar datos", ""}."Inicio" -> [w582]
                      tunnel: w576 -> [w579]
                      stop <- w581 stop-if-true
                      n286 = case shown="\"Tomar datos\"" w582 {
                        tunnel: [w583 w594] -> w580
                        tunnel: w579 -> [_ w589]
                        frame "Inicio", Default {
                          # "Se chequea si el usuario ha presionado el boton de comenzar el experimento. Si no lo ha hecho, se queda en este estado (0).\n Cuando lo presiona, pasa al estado de adquirir datios (1) ."
                          n287 = Select(t=enum16{"Inicio", "Tomar datos", ""}."Tomar datos", s="Iniciar experimento", f=enum16{"Inicio", "Tomar datos", ""}."Inicio") -> (s? t:f=w583:enum16{"Inicio", "Tomar datos", ""})
                        }
                        frame "Tomar datos" {
                          n288 = flat-sequence {
                            tunnel: [w687] -> w593
                            tunnel: [w686] -> w592
                            tunnel: [w685] -> w591
                            tunnel: [w684] -> w590
                            tunnel: w589 -> [w678]
                            tunnel: [w661] -> w588
                            tunnel: [w641] -> w587
                            tunnel: w593 -> [w994]
                            tunnel: w592 -> [w993]
                            tunnel: w591 -> [w992]
                            tunnel: w590 -> [w991]
                            tunnel: w588 -> [w988]
                            tunnel: w587 -> [w989]
                            tunnel: [enum16{"Inicio", "Tomar datos", ""}."Inicio"] -> w594
                            frame #0 {
                              w598 = 10123 items=["Finite Samples"=10178, "Continuous Samples"=10123, "Hardware Timed Single Point"=12522] ("sample mode")
                              w602 = 10083 items=["Default"=-1, "RSE"=10083, "NRSE"=10078, "Differential"=10106, "Pseudodifferential"=12529] ("input terminal configuration")
                              w627 = u16 0 items=["None", "Last Bit", "TermChar", "Break"] ("Serial Settings:End Mode for Writes")
                              w628 = u16 2 items=["None", "Last Bit", "TermChar"] ("Serial Settings:End Mode for Reads")
                              w652 = u16 0 items=["None", "Last Bit", "TermChar", "Break"] ("Serial Settings:End Mode for Writes")
                              w653 = u16 2 items=["None", "Last Bit", "TermChar"] ("Serial Settings:End Mode for Reads")
                              w676 = 100  # max queue size
                              # "[9] Se unen en una sola matriz los vectores de tiempo, distancia, potencia derecha y potencia izquierda."
                              # "[9]"
                              # "[12] Se unen en una sola matriz, los vectores de  tiempo de la señal EMG, amplitud de la señal EMG, tiempo de potencia óptica, distancia, potencia óptica derecha y potencia óptica izquierda, en ese orden."
                              # "[8]"
                              # "[7]"
                              # "[6]"
                              # "[5]"
                              # "Se usan registros de desplazamiento para concatenar en un solo vector los datos que se obtienen en cada iteracion. Así en \n[1] Se guarda la potencia del lente derecho.\n[2] Por medio de variables locales, se guarda la distancia que se obtuvo en el bloque de distancia.\n[3]  Por medio de variables locales, se guarda la potencia del lente izquierdo que se obtuvo en el bloque de control de potencia del lente izquierdo.\n[4] Se guarda el tiempo actual.\n[5] Se pasa el vector de de potencia derecha a variable a string con 2 cifras significativas. \n[6] Se ajusta el vector del tiempo para que se muestre un tiempo relativo, es decir, en donde el primer dato sea 0 y en los demas se aumente un dt.  Además, se pasa el vector a variable a string con 5 cifras significativas.\n[7] Se pasa el vector de de distancia a variable a string con 0 cifras significativas. \n[8] Se pasa el vector de de potencia izquierda a variable a string con 2 cifras significativas."
                              # "En esta cola se guarda los datos de la señal EMG\nEn el bloque de adquisición los añade al adquirirlos y  en el de procesamiento los elimina al procesarlos ."
                              # "Initialize VISA port with correct parameters"
                              # "Initialize VISA port with correct parameters"
                              # "Close VISA port after program stop. Otherwise this port is blocked."
                              # "Se adquiere la señal del circuito de adquisicion, en donde se define la frecuencia de muestreo y el factor de decimacion.\n[1] Se inicializa el canal de adquisicion\n[2] Se ajusta el canal para que lea muestras continuas y apartir de estas prooduzca waveform data.\n[3]  Se obtiene los datos de la señal: la amplitud Y, el tiempo de inicio y el delta t.\n[4] Se decima el vector de amplitud. \n[5] Se usan registros de desplazamiento para concatenenar en un solo vector los datos de la amplitud que se obtienen en cada iteración. \n[6] Se obtiene el vector del tiempo."
                              # "[11] Los vectores de amplitud y tiempo se transforman a formato texto con 4 y 5 cifras significativas respectivamente y se unen para formar un vector de 2 columnas."
                              # "[9] Se ajusta el vector del tiempo para que se muestre un tiempo relativo, es decir, en donde el primer dato sea 0 y en los demas se aumente un dt. \n[10] Se extrae el primer elemento del vector ya que este siempre es 0 y no aporta información"
                              # "[12]"
                              # "[11]"
                              # "[10]"
                              # "[9]"
                              # "[8] Se guarda la fecha/hora en que se inicio el experimento"
                              # "[7] Se usan registros de desplazamiento para concatenar en un solo vector los datos del tiempo que se obtienen en cada iteracion."
                              # "[1]"
                              n289 = local read "error in (no error)"() -> (w648:errorcluster)
                              n290 = local read "VISA resource name"() -> (w647:string)
                              n291 = local read "VISA resource name 2"() -> (w623:string)
                              n292 = call-poly "VISA Configure Serial Port"("VISA resource name"=w647, "timeout (10sec)"=u32 2000, "Enable Termination\nChar (T)"=FALSE ("Enable Termination\nChar (T)"), "baud rate (9600)"=u32 115200, "error in (no error)"=w648) -> ("VISA resource name out"=w657:refnum<visa-resource-name>, "error out"=w655:errorcluster)  [unwired: 9 in]
                              n293 = call-poly "VISA Configure Serial Port"("VISA resource name"=w623, "timeout (10sec)"=u32 2000, "Enable Termination\nChar (T)"=FALSE ("Enable Termination\nChar (T)"), "baud rate (9600)"=u32 115200, "error in (no error)"="error in (no error) 5") -> ("VISA resource name out"=w632:refnum<visa-resource-name>, "error out"=w630:errorcluster)  [unwired: 9 in]
                              n294 = property class="Instr"(reference=w657, error in=w655, "TermChar"=u8 10 ("Message Based Settings:Termination Character"), "ASRL End In"=w653, "ASRL End Out"=w652) -> (reference out=w656:refnum<visa-resource-name>, error out=w654:errorcluster)
                              n295 = property class="Instr"(reference=w632, error in=w630, "TermChar"=u8 10 ("Message Based Settings:Termination Character"), "ASRL End In"=w628, "ASRL End Out"=w627) -> (reference out=w631:refnum<visa-resource-name>, error out=w629:errorcluster)
                              n296 = VISA Set I/O Buffer Size(VISA resource name=w656, error in (no error)=w654) -> (VISA resource name out=w650:refnum<visa-resource-name>, error out=w649:errorcluster)  [unwired: 2 in]
                              n297 = VISA Set I/O Buffer Size(VISA resource name=w631, error in (no error)=w629) -> (VISA resource name out=w625:refnum<visa-resource-name>, error out=w624:errorcluster)  [unwired: 2 in]
                              n298 = VISA Flush I/O Buffer(VISA resource name=w650, error in (no error)=w649) -> (VISA resource name out=w646:refnum<visa-resource-name>, error out=w645:errorcluster)  [unwired: 1 in]
                              n299 = call-poly <vilib>:"DAQmx Create Virtual Channel.vi"("input terminal configuration"=w602, "physical channels"=tag "Dev1/ai0") -> ("task out"=w601:refnum<k21>, "error out"=w600:errorcluster)  [unwired: 12 in]
                              n300 = VISA Flush I/O Buffer(VISA resource name=w625, error in (no error)=w624) -> (VISA resource name out=w621:refnum<visa-resource-name>, error out=w620:errorcluster)  [unwired: 1 in]
                              n301 = invoke on="Parar adquisicion" class="Bool (strict)" method="Reinit To Default"() -> ()  [unwired: 3 in, 3 out]
                              n302 = Obtain Queue(max queue size (-1, unlimited)=w676, element data type="Cola tipo 2") -> (queue out=w675:refnum<queue>)  [unwired: 3 in, 2 out]
                              n303 = Enqueue Element(queue=w678, element=0.0) -> (queue out=w681:refnum<queue>)  [unwired: 2 in, 2 out]
                              n304 = call-poly <vilib>:"DAQmx Timing.vi"("task/channels in"=w601, "sample mode"=w598, "samples per channel"=1000, "rate"=1000.0, "error in"=w600) -> ("task out"=w596:refnum<k21>, "error out"=w595:errorcluster)  [unwired: 9 in]
                              n305 = call <vilib>:"DAQmx Start Task.vi"("task/channels in"=w596, "error in"=w595) -> ("task out"=w700:refnum<k21>, "error out"=w701:errorcluster)  [unwired: 12 in]
                              n306 = local read "tamaño buffer"() -> (w699:i32)
                              n307 = case shown="No Error" w620 {
                                tunnel: w620 -> [w724 w781]
                                tunnel: w621 -> [w723 w782]
                                tunnel: [w722 w781] -> w607
                                tunnel: [w721 w782] -> w606
                                tunnel: [w711 dbl[] [-30.0]] -> _
                                frame No Error {
                                w720 = 2 ("length (rest)")
                                # "Bloque de control del izquierdo. Se explica en el caso 0 de visualziación general"
                                # "Initialize Lens Driver"
                                n308 = local read "Calibration"() -> (w712:T2)
                                n309 = for {
                                tunnel: w723 -> [w778]
                                tunnel: [w775] -> w715
                                tunnel: string[] ["Start", "MwDA", "CrMA00", "CrMB00", "CrUA00", "CrUB00", "CrLA00", "CrLB00", "PwTA\u0002Ð\u0001@"] -> [w773] mode=indexing
                                tunnel: [w772] -> w714
                                shift-right: [w776] -> w716
                                shift-left: w712 -> [w777]
                                shift-right: [w774] -> w717
                                shift-left: w724 -> [w779]
                                n310 = call "write read Lens Driver.vi"("VISA resource name"=w778, "command"=w773, "Calibration"=w777, "error in (no error)"=w779) -> ("VISA resource name out"=w775:refnum<visa-resource-name>, "Calibration 2"=w776:T2, "Data"=w772:string, "error out"=w774:errorcluster)  [unwired: 4 in, 4 out]
                                }
                                n311 = String Subset(string=w714, offset (0)=w720, length (rest)=w720) -> (substring=w718:string)
                                n312 = Type Cast(type=u16 0 ("length (rest)"), x=w718) -> (*(type *) &x=w713:u16)
                                n313 = local write "ID"(w713) -> ()
                                n314 = while {
                                tunnel: [w729] -> w722
                                tunnel: [w730] -> w721
                                tunnel: w717 -> [w735]
                                tunnel: w716 -> [w734]
                                tunnel: w715 -> [w733]
                                shift-right: [w726] -> w711
                                shift-left: _ -> [w727]
                                stop <- w728 stop-if-true
                                # "When Send command is true, Current Ch A is sent to the Lens Driver, in the correct format. If answer exists it is displayed in Data. The update rate of the while loop is 2ms."
                                n315 = case shown="True" TRUE ("Send command") {
                                tunnel: [w741 w764] -> w729
                                tunnel: w735 -> [w741 w763]
                                tunnel: w734 -> [_ w744]
                                tunnel: w733 -> [w740 w762]
                                tunnel: [w740 w755] -> w730
                                tunnel: [dbl[] [-20.0] w754] -> w726
                                tunnel: w727 -> [_ w753]
                                frame False {
                                }
                                frame True {
                                n316 = local read "Potencia inicial lente izquierdo"() -> (w752:dbl)
                                n317 = local read "DPT dif."() -> (w751:dbl)
                                n318 = Add(x=w751, y=w752) -> (x+y=w747:dbl)
                                n319 = Absolute Value(x=w747) -> (abs(x)=w749:dbl)
                                n320 = Greater Or Equal?(x=6.0, y=w749) -> (x >= y?=w748:bool)
                                n321 = case shown="False" w748 {
                                tunnel: w747 -> [w767 w771]
                                tunnel: [w765 w771] -> w745
                                frame False {
                                n322 = Greater Or Equal?(x=u16 0, y=w767) -> (x >= y?=w768:bool)
                                n323 = case shown="False" w768 {
                                tunnel: [i16 6 ("x") i16 -6 ("x")] -> w765
                                frame False {
                                }
                                frame True {
                                }
                                }
                                }
                                frame True {
                                }
                                }
                                "Potencia izquierdo" <- w745
                                n324 = Unbundle By Name(w744) -> ("Max Current A"=w743:dbl)
                                n325 = call "potencia a corriente.vi"("Max current A"=w743, "Potencia"=w745) -> ("Corriente"=w746:dbl)
                                n326 = To Word Integer(number=w746) -> (16bit integer=w761:i16)
                                n327 = Type Cast(x=w761) -> (*(type *) &x=w760:string)  [unwired: 1 in]
                                n328 = Concatenate Strings("Aw", w760) -> (w757:string)
                                n329 = local write "Command to Port"(w757) -> ()
                                n330 = call "write read Lens Driver.vi"("VISA resource name"=w762, "command"=w757, "Calibration"=w744, "error in (no error)"=w763) -> ("VISA resource name out"=w755:refnum<visa-resource-name>, "Calibration 2"=w759:T2, "OK"=w758:bool, "Data"=w756:string, "error out"=w764:errorcluster)  [unwired: 4 in, 3 out]
                                n331 = local write "VISA resource name 2"(w755) -> ()
                                n332 = local write "Calibration 2"(w759) -> ()
                                n333 = local write "Data"(w756) -> ()
                                n334 = local write "OK"(w758) -> ()
                                n335 = Build Array (concatenate)(w753, w745) -> (w754:dbl[])
                                }
                                }
                                n336 = Wait Until Next ms Multiple(millisecond multiple=u32 10) -> ()  [unwired: 1 out]
                                n337 = local read "Parar adquisicion"() -> (w728:bool)
                                n338 = event shown="[0] \"Restablecer Iniciales\": Value Change" {
                                selector: _ -> [_ _]
                                dyn-events: _ -> [_ _]
                                timeout: 100 -> [_ _]
                                event "Restablecer Iniciales": Value Change {
                                n339 = event-data() -> ()  [unwired: 1 in, 3 out]
                                n340 = local read "Potencia inicial lente izquierdo"() -> (w736:dbl)
                                n341 = local read "Potencia inicial lente derecho"() -> (w737:dbl)
                                n342 = local write "Potencia izquierdo"(w736) -> ()
                                n343 = local write "Potencia derecho"(w737) -> ()
                                n344 = local write "DPT dif."(0.0 ("DPT dif.")) -> ()
                                }
                                event Timeout {
                                n345 = event-data() -> ()  [unwired: 1 in, 3 out]
                                }
                                }
                                }
                                }
                                frame Error {
                                }
                              }
                              n346 = case shown="No Error" w645 {
                                tunnel: w645 -> [w804 w900]
                                tunnel: w646 -> [w803 w901]
                                tunnel: [w802 w900] -> w673
                                tunnel: [w801 w901] -> w672
                                tunnel: [w790 dbl[] [-1.0]] -> w665
                                tunnel: [w789 dbl[] [-30.0]] -> w613
                                tunnel: [w788 u32[] [0]] -> w643
                                tunnel: [w786 dbl[] [-30.0]] -> w616
                                frame No Error {
                                w800 = 2 ("length (rest)")
                                # "Bloque de control del lente derecho. Se explica en el caso 0 de visualziación general"
                                # "Initialize Lens Driver"
                                n347 = local read "Calibration"() -> (w792:T2)
                                n348 = for {
                                tunnel: w803 -> [w894]
                                tunnel: [w891] -> w795
                                tunnel: string[] ["Start", "MwDA", "CrMA00", "CrMB00", "CrUA00", "CrUB00", "CrLA00", "CrLB00", "PwTA\u0002Ð\u0001@"] -> [w889] mode=indexing
                                tunnel: [w888] -> w794
                                shift-right: [w892] -> w796
                                shift-left: w792 -> [w893]
                                shift-right: [w890] -> w797
                                shift-left: w804 -> [w895]
                                n349 = call "write read Lens Driver.vi"("VISA resource name"=w894, "command"=w889, "Calibration"=w893, "error in (no error)"=w895) -> ("VISA resource name out"=w891:refnum<visa-resource-name>, "Calibration 2"=w892:T2, "Data"=w888:string, "error out"=w890:errorcluster)  [unwired: 4 in, 4 out]
                                }
                                n350 = String Subset(string=w794, offset (0)=w800, length (rest)=w800) -> (substring=w798:string)
                                n351 = Type Cast(type=u16 0 ("length (rest)"), x=w798) -> (*(type *) &x=w793:u16)
                                n352 = local write "ID"(w793) -> ()
                                n353 = while {
                                tunnel: [w822] -> w802
                                tunnel: [w823] -> w801
                                tunnel: w797 -> [w828]
                                tunnel: w796 -> [w827]
                                tunnel: w795 -> [w826]
                                shift-right: [w809] -> w790
                                shift-left: dbl[] [0.0] -> [w810]
                                shift-right: [w817] -> w789
                                shift-left: dbl[] [0.0] -> [w820]
                                shift-right: [w816] -> w788
                                shift-left: u32[] [0] -> [w819]
                                shift-right: [w807] -> w786
                                shift-left: dbl[] [0.0] -> [w806]
                                stop <- w821 stop-if-true
                                # "[4]"
                                # "[3]"
                                # "[2]"
                                # "When Send command is true, Current Ch A is sent to the Lens Driver, in the correct format. If answer exists it is displayed in Data. The update rate of the while loop is 2ms."
                                n354 = Wait Until Next ms Multiple(millisecond multiple=u32 10) -> ()  [unwired: 1 out]
                                n355 = case shown="True" TRUE ("Send command") {
                                tunnel: [w835 w854] -> w822
                                tunnel: w828 -> [w835 w853]
                                tunnel: w827 -> [_ w838]
                                tunnel: w826 -> [w834 w852]
                                tunnel: [w834 w844] -> w823
                                tunnel: [dbl[] [-20.0] w843] -> w817
                                tunnel: w820 -> [_ w842]
                                frame False {
                                }
                                frame True {
                                # "[1]"
                                n356 = local read "number"() -> (w849:u32)
                                n357 = local read "Potencia inicial lente derecho"() -> (w841:dbl)
                                n358 = case shown="2" w849 {
                                tunnel: [w855 w864 w879] -> w840
                                tunnel: w841 -> [w857 w859 w874]
                                tunnel: w841 -> [_ w858 w873]
                                frame 0, Default {
                                n359 = local read "DPT dif."() -> (w856:dbl)
                                n360 = Add(x=w857, y=w856) -> (x+y=w855:dbl)
                                }
                                frame 1 {
                                n361 = local read "DPT dif."() -> (w860:dbl)
                                n362 = Add(x=w859, y=w860) -> (x+y=w861:dbl)
                                n363 = Less Or Equal?(x=w861, y=6.0) -> (x <= y?=w863:bool)
                                n364 = case shown="True" w863 {
                                tunnel: [w866 w870] -> w864
                                tunnel: w858 -> [w865 w869]
                                frame False {
                                n365 = local read "DPT dif."() -> (w867:dbl)
                                n366 = Add(x=w865, y=w867) -> (x+y=w866:dbl)
                                }
                                frame True {
                                n367 = local read "DPT dif."() -> (w871:dbl)
                                n368 = local read "Incremento"() -> (w868:dbl)
                                n369 = Add(x=w871, y=w868) -> (x+y=w872:dbl)
                                n370 = local write "DPT dif."(w872) -> ()
                                n371 = Add(x=w869, y=w872) -> (x+y=w870:dbl)
                                }
                                }
                                }
                                frame 2 {
                                n372 = local read "DPT dif."() -> (w878:dbl)
                                n373 = Add(x=w878, y=w874) -> (x+y=w875:dbl)
                                n374 = Greater Or Equal?(x=w875, y=-6.0) -> (x >= y?=w876:bool)
                                n375 = case shown="True" w876 {
                                tunnel: [w881 w885] -> w879
                                tunnel: w873 -> [w880 w884]
                                frame False {
                                n376 = local read "DPT dif."() -> (w882:dbl)
                                n377 = Add(x=w880, y=w882) -> (x+y=w881:dbl)
                                }
                                frame True {
                                n378 = local read "DPT dif."() -> (w887:dbl)
                                n379 = local read "Incremento"() -> (w883:dbl)
                                n380 = Subtract(x=w887, y=w883) -> (x-y=w886:dbl)
                                n381 = local write "DPT dif."(w886) -> ()
                                n382 = Add(x=w884, y=w886) -> (x+y=w885:dbl)
                                }
                                }
                                }
                                }
                                "Potencia derecho" <- w840
                                n383 = Unbundle By Name(w838) -> ("Max Current A"=w837:dbl)
                                n384 = call "potencia a corriente.vi"("Max current A"=w837, "Potencia"=w840) -> ("Corriente"=w839:dbl)
                                n385 = To Word Integer(number=w839) -> (16bit integer=w851:i16)
                                n386 = Type Cast(x=w851) -> (*(type *) &x=w850:string)  [unwired: 1 in]
                                n387 = Concatenate Strings("Aw", w850) -> (w846:string)
                                n388 = local write "Command to Port"(w846) -> ()
                                n389 = call "write read Lens Driver.vi"("VISA resource name"=w852, "command"=w846, "Calibration"=w838, "error in (no error)"=w853) -> ("VISA resource name out"=w844:refnum<visa-resource-name>, "Calibration 2"=w848:T2, "OK"=w847:bool, "Data"=w845:string, "error out"=w854:errorcluster)  [unwired: 4 in, 3 out]
                                n390 = local write "VISA resource name out"(w844) -> ()
                                n391 = local write "Calibration 2"(w848) -> ()
                                n392 = local write "Data"(w845) -> ()
                                n393 = local write "OK"(w847) -> ()
                                n394 = Build Array (concatenate)(w842, w840) -> (w843:dbl[])
                                }
                                }
                                n395 = local read "Parar adquisicion"() -> (w821:bool)
                                n396 = local read "Potencia izquierdo"() -> (w805:dbl)
                                n397 = local read "Distancia"() -> (w818:u32)
                                n398 = property on="Potencia optica y distancia" class="WFChart (strict)"("YScale.ScaleFit"="Auto scale Y") -> ()  [unwired: 2 in, 2 out]
                                n399 = Get Date/Time In Seconds() -> (seconds since 1Jan1904=w811:timestamp)
                                n400 = To Double Precision Float(number=w811) -> (double precision float=w808:dbl)
                                n401 = property on="Potencia optica y distancia" class="WFChart (strict)"("XScale.ScaleFit"="Auto scale X") -> ()  [unwired: 2 in, 2 out]
                                n402 = Build Array (concatenate)(w810, w808) -> (w809:dbl[])
                                n403 = case shown="0, Default" "Auto scale Y" {
                                frame 0, Default {
                                n404 = property on="Potencia optica y distancia" class="WFChart (strict)"("YScale.Maximum"="Escala Y max") -> ()  [unwired: 2 in, 2 out]
                                n405 = property on="Potencia optica y distancia" class="WFChart (strict)"("YScale.Minimum"="Escala Y min") -> ()  [unwired: 2 in, 2 out]
                                }
                                frame 1 {
                                }
                                }
                                n406 = Build Array (concatenate)(w806, w805) -> (w807:dbl[])
                                n407 = Build Array (concatenate)(w819, w818) -> (w816:u32[])
                                n408 = case shown="0, Default" "Auto scale X" {
                                frame 0, Default {
                                n409 = property on="Potencia optica y distancia" class="WFChart (strict)"("XScale.Maximum"="Escala X max") -> ()  [unwired: 2 in, 2 out]
                                n410 = property on="Potencia optica y distancia" class="WFChart (strict)"("XScale.Minimum"="Escala X min") -> ()  [unwired: 2 in, 2 out]
                                }
                                frame 1 {
                                }
                                }
                                n411 = Build Array(w817, w816) -> (w815:dbl[][])
                                n412 = Transpose 2D Array(2D array=w815) -> (transposed array=→"Potencia optica y distancia":dbl[][])
                                }
                                }
                                frame Error {
                                }
                              }
                              n413 = while {
                                tunnel: w681 -> [w933]
                                shift-right: [w935] -> _
                                shift-left: dbl[] [0.0] -> [w941]
                                shift-right: [w934] -> _
                                shift-left: u32[] [0] -> [w936]
                                tunnel: [w933] -> w679
                                tunnel: w675 -> [w925]
                                stop <- w924 stop-if-true
                                # "Bloque de procesamiento.  Se explica en el caso 0 de visualización general"
                                n414 = local read "WL"() -> (w932:dbl)
                                n415 = local read "Parar adquisicion"() -> (w924:bool)
                                n416 = local read "Limite superior WL"() -> (w929:dbl)
                                n417 = call "waveform_length.vi"("WL"=w932, "Cola WL"=w933, "Datos entrada"=w925) -> ("WL 2"=w940:dbl)
                                n418 = local read "Limite inferior WL"() -> (w931:dbl)
                                n419 = local write "WL"(w940) -> ()
                                n420 = Build Array (concatenate)(w941, w940) -> (w935:dbl[])
                                n421 = In Range and Coerce(upper limit=w929, x=w940, lower limit=w931) -> (In Range?=w938:bool)  [unwired: 1 out]
                                n422 = Greater?(x=w940, y=w929) -> (0:w939:bool)
                                n423 = local read "Escala autom. X"() -> (w926:u8)
                                n424 = local read "Escala autom. Y"() -> (w927:u8)
                                n425 = Build Array(w939, w938) -> (w937:bool[])
                                n426 = Boolean Array To Number(Boolean array=w937) -> (number=w930:u32)
                                n427 = local write "number"(w930) -> ()
                                n428 = Build Array (concatenate)(w936, w930) -> (w934:u32[])
                                n429 = Build Array(w935, w934) -> (w928:dbl[][])
                                n430 = Transpose 2D Array(2D array=w928) -> (transposed array=w923:dbl[][])
                                n431 = local write "Waveform length"(w923) -> ()
                                n432 = property on="Waveform length" class="WFChart (strict)"("XScale.ScaleFit"=w926) -> ()  [unwired: 2 in, 2 out]
                                n433 = property on="Waveform length" class="WFChart (strict)"("YScale.ScaleFit"=w927) -> ()  [unwired: 2 in, 2 out]
                                n434 = case shown="0, Default" w927 {
                                frame 0, Default {
                                n435 = local read "Maximo escala Y"() -> (w945:dbl)
                                n436 = local read "Minimo escala Y"() -> (w944:dbl)
                                n437 = property on="Waveform length" class="WFChart (strict)"("YScale.Maximum"=w945) -> ()  [unwired: 2 in, 2 out]
                                n438 = property on="Waveform length" class="WFChart (strict)"("YScale.Minimum"=w944) -> ()  [unwired: 2 in, 2 out]
                                }
                                frame 1 {
                                }
                                }
                                n439 = case shown="0, Default" w926 {
                                frame 0, Default {
                                n440 = local read "Minimo escala X"() -> (w943:dbl)
                                n441 = local read "Maximo escala X"() -> (w942:dbl)
                                n442 = property on="Waveform length" class="WFChart (strict)"("XScale.Minimum"=w943) -> ()  [unwired: 2 in, 2 out]
                                n443 = property on="Waveform length" class="WFChart (strict)"("XScale.Maximum"=w942) -> ()  [unwired: 2 in, 2 out]
                                }
                                frame 1 {
                                }
                                }
                              }
                              n444 = while {
                                tunnel: w700 -> [w978]
                                tunnel: w699 -> [w975]
                                tunnel: [w976] -> w689
                                shift-right: [w973] -> w688
                                shift-left: w701 -> [w977]
                                tunnel: [w968] -> w709
                                shift-right: [w967] -> w686
                                shift-left: _ -> [w966]
                                shift-right: [w957] -> w691
                                shift-left: dbl[] [0.0] -> [w962]
                                shift-right: [w958] -> w696
                                shift-left: dbl[] [0.0] -> [w959]
                                tunnel: w675 -> [w950]
                                i -> [w969]
                                stop <- w972 stop-if-true
                                w971 = 10.0  # timeout (s)
                                # "[7]"
                                # "[6]"
                                # "[5]"
                                # "[4]"
                                # "[3]"
                                # "[2]"
                                n445 = local read "Escala automatica X"() -> (w948:u8)
                                n446 = local read "Escala automatica Y"() -> (w947:u8)
                                n447 = property on="Senal EMG" class="WFGraph (strict)"("XScale.ScaleFit"=w948) -> ()  [unwired: 2 in, 2 out]
                                n448 = case shown="0, Default" w948 {
                                frame 0, Default {
                                n449 = local read "X Scale.Range:Increment"() -> (w981:dbl)
                                n450 = local read "X Scale.Range:Minimum"() -> (w982:dbl)
                                n451 = local read "X Scale.Range:Maximum"() -> (w983:dbl)
                                n452 = property on="Senal EMG" class="WFGraph (strict)"("XScale.Increment"=w981) -> ()  [unwired: 2 in, 2 out]
                                n453 = property on="Senal EMG" class="WFGraph (strict)"("XScale.Minimum"=w982) -> ()  [unwired: 2 in, 2 out]
                                n454 = property on="Senal EMG" class="WFGraph (strict)"("XScale.Maximum"=w983) -> ()  [unwired: 2 in, 2 out]
                                }
                                frame 1 {
                                }
                                }
                                n455 = local read "Parar adquisicion"() -> (w953:bool)
                                n456 = call-poly <vilib>:"DAQmx Read.vi"("task/channels in"=w978, "number of samples per channel"=w975, "timeout"=w971, "error in"=w977) -> ("task out"=w976:refnum<k21>, "data"=w963:waveform(dbl)[], "error out"=w973:errorcluster)  [unwired: 9 in]
                                n457 = Unbundle By Name(w973) -> ("status"=w974:bool)
                                n458 = Or(x=w974, y=w953) -> (x .or. y?=w972:bool)
                                n459 = property on="Senal EMG" class="WFGraph (strict)"("YScale.ScaleFit"=w947) -> ()  [unwired: 2 in, 2 out]
                                n460 = local write "Senal EMG"(w963) -> ()
                                n461 = case shown="0, Default" w947 {
                                frame 0, Default {
                                n462 = local read "Y Scale.Range:Maximum"() -> (w980:dbl)
                                n463 = local read "Y Scale.Range:Minimum"() -> (w979:dbl)
                                n464 = property on="Senal EMG" class="WFGraph (strict)"("YScale.Minimum"=w979) -> ()  [unwired: 2 in, 2 out]
                                n465 = property on="Senal EMG" class="WFGraph (strict)"("YScale.Maximum"=w980) -> ()  [unwired: 2 in, 2 out]
                                }
                                frame 1 {
                                }
                                }
                                n466 = call-poly <vilib>:"Index Waveform Array.vi"("index"=0, "waveform array"=w963) -> ("waveform"=w961:waveform(dbl))  [unwired: 8 in, 1 out]
                                n467 = Unbundle By Name(w961) -> ("Y"=w951:dbl[], "t0"=w968:timestamp)  [unwired: 1 out]
                                n468 = call-poly <vilib>:"Decimate (continuous).vi"("averaging"=TRUE, "decimating factor"="factor decimacion", "X"=w951) -> ("Decimated Array"=w946:dbl[])  [unwired: 7 in, 1 out]
                                n469 = Lossy Enqueue Element(queue=w950, element=w946) -> ()  [unwired: 1 in, 4 out]
                                n470 = Build Array (concatenate)(w962, w946) -> (w957:dbl[])
                                n471 = case shown="1" w969 {
                                tunnel: w968 -> [_ w987]
                                tunnel: [w985 w986] -> w967
                                tunnel: w966 -> [w985 _]
                                frame 0, Default {
                                }
                                frame 1 {
                                # "[8]"
                                n472 = Format Date/Time String(seconds (now)=w987) -> (date/time string=w986:string)  [unwired: 2 in]
                                }
                                }
                                n473 = local read "factor decimacion"() -> (w954:i32)
                                n474 = call-poly <vilib>:"Get Waveform Time Array.vi"("waveform in"=w961) -> ("X array"=w960:timestamp[])  [unwired: 9 in, 1 out]
                                n475 = event shown="[0] \"Ganancia\": Value Change" {
                                selector: _ -> [_ _]
                                dyn-events: _ -> [_ _]
                                timeout: 1 -> [_ _]
                                tunnel: "Ganancia" -> [w984 _]
                                event "Ganancia": Value Change {
                                n476 = event-data() -> ()  [unwired: 1 in, 4 out]
                                n477 = call "Ganancia programable.vi"("MOSI data"=w984) -> ()
                                }
                                event Timeout {
                                n478 = event-data() -> ()  [unwired: 1 in, 3 out]
                                }
                                }
                                n479 = To Double Precision Float(number=w960) -> (double precision float=w956:dbl[])
                                n480 = call-poly <vilib>:"Decimate (single shot).vi"("decimating factor"=w954, "X"=w956) -> ("Decimated Array"=w955:dbl[])  [unwired: 8 in, 1 out]
                                n481 = Build Array (concatenate)(w959, w955) -> (w958:dbl[])
                              }
                              n482 = call <vilib>:"DAQmx Clear Task.vi"("task in"=w689, "error in"=w688) -> ()  [unwired: 13 in, 1 out]
                              n483 = Index Array(array=w696, index=1) -> (element=w695:dbl)
                              n484 = Flush Queue(queue=w679) -> ()  [unwired: 1 in, 3 out]
                              n485 = Subtract(x=w696, y=w695) -> (x-y=w693:dbl[])
                              n486 = Delete From Array(array=w691, index=0) -> (array with subset deleted=w704:dbl[])  [unwired: 1 in, 1 out]
                              n487 = while {
                                shift-right: [w902] -> _
                                shift-left: _ -> [w903]
                                stop <- w907 stop-if-true
                                # "Este bloque adquiere la distancia (se explica en el caso 0 (visualizacion general)"
                                n488 = call "meididor de distancia archivo adicional.vi"() -> ("error out"=w910:errorcluster, "task out"=w911:refnum<k21>)  [unwired: 10 in]
                                n489 = call "DAQ Assistant2"("timeout (s)"=0.05) -> ("data"=w920:dynamicdata, "error out"=w908:errorcluster)  [unwired: 16 in, 1 out]
                                n490 = call <vilib>:"DAQmx Start Task.vi"("task/channels in"=w911, "error in"=w910) -> ("task out"=w914:refnum<k21>, "error out"=w915:errorcluster)  [unwired: 12 in]
                                n491 = call <vilib>:"DAQmx Is Task Done.vi"("task/channels in"=w914, "error in"=w915) -> ("task out"=w912:refnum<k21>, "error out"=w913:errorcluster)  [unwired: 11 in, 1 out]
                                n492 = Wait (ms)(milliseconds to wait=u32 200) -> ()  [unwired: 1 out]
                                n493 = call <vilib>:"Clear Errors.vi"("error in (no error)"=w908) -> ()  [unwired: 5 in, 2 out]
                                n494 = local read "Parar adquisicion"() -> (w907:bool)
                                n495 = call <vilib>:"DAQmx Clear Task.vi"("task in"=w912, "error in"=w913) -> ()  [unwired: 13 in, 1 out]
                                n496 = Multiply(x=1000000.0, y=w920) -> (x*y=w918:dynamicdata)
                                n497 = Divide(x=w918, y=58.0) -> (x/y=w904:dynamicdata)
                                n498 = Equal?(x=w904, y=0.0) -> (x = y?=w906:dynamicdata)
                                n499 = case shown="True" w906 {
                                tunnel: [w921 w922] -> w902
                                tunnel: w904 -> [w921 _]
                                tunnel: w903 -> [_ w922]
                                frame False {
                                }
                                frame True {
                                }
                                }
                                n500 = local write "Distancia"(w902) -> ()
                              }
                              n501 = Delete From Array(array=w693, index=0) -> (array with subset deleted=w703:dbl[])  [unwired: 1 in, 1 out]
                              n502 = local read "path"() -> (w687:path)
                              n503 = Format Date/Time String(seconds (now)=w709) -> (date/time string=w685:string)  [unwired: 2 in]
                              n504 = Number To Fractional String(use system decimal point (T)=FALSE, number=w704, precision (6)=i16 4) -> (F-format string=w639:string[])  [unwired: 1 in]
                              n505 = Number To Fractional String(use system decimal point (T)=FALSE, number=w703, precision (6)=i16 5) -> (F-format string=w640:string[])  [unwired: 1 in]
                              n506 = Build Array(w640, w639) -> (w702:string[][])
                              n507 = Transpose 2D Array(2D array=w702) -> (transposed array=w684:string[][])
                              n508 = Delete From Array(array=w613, index=0) -> (array with subset deleted=w612:dbl[])  [unwired: 1 in, 1 out]
                              n509 = Delete From Array(array=w643, index=0) -> (array with subset deleted=w609:u32[])  [unwired: 1 in, 1 out]
                              n510 = Index Array(array=w665, index=1) -> (element=w670:dbl)
                              n511 = Delete From Array(array=w616, index=0) -> (array with subset deleted=w615:dbl[])  [unwired: 1 in, 1 out]
                              n512 = VISA Close(VISA resource name=w606, error in (no error)=w607) -> (error out=w605:errorcluster)
                              n513 = Subtract(x=w665, y=w670) -> (x-y=w664:dbl[])
                              n514 = Number To Fractional String(use system decimal point (T)=FALSE, number=w612, precision (6)=i16 2) -> (F-format string=w636:string[])  [unwired: 1 in]
                              n515 = VISA Close(VISA resource name=w672, error in (no error)=w673) -> (error out=w674:errorcluster)
                              n516 = call <vilib>:"Simple Error Handler.vi"("error in (no error)"=w605) -> ("error out"=w604:errorcluster)  [unwired: 4 in, 4 out]
                              n517 = Number To Fractional String(number=w609, precision (6)=i16 0) -> (F-format string=w637:string[])  [unwired: 2 in]
                              n518 = Delete From Array(array=w664, index=0) -> (array with subset deleted=w669:dbl[])  [unwired: 1 in, 1 out]
                              n519 = call <vilib>:"Simple Error Handler.vi"("error in (no error)"=w674) -> ("error out"=w671:errorcluster)  [unwired: 4 in, 4 out]
                              n520 = Number To Fractional String(use system decimal point (T)=FALSE, number=w615, precision (6)=i16 2) -> (F-format string=w617:string[])  [unwired: 1 in]
                              n521 = local write "error out"(w671) -> ()
                              n522 = local write "error out"(w604) -> ()
                              n523 = Number To Fractional String(use system decimal point (T)=FALSE, number=w669, precision (6)=i16 5) -> (F-format string=w638:string[])  [unwired: 1 in]
                              n524 = Build Array(w640, w639, w638, w637, w636, w617) -> (w610:string[][])
                              n525 = Transpose 2D Array(2D array=w610) -> (transposed array=w641:string[][])
                              n526 = Build Array(w638, w637, w636, w617) -> (w661:string[][])
                            }
                            frame #1 {
                              # "[13]"
                              # "[13] En esta case structure, se decide que datos se van a guardar. Esto lo hace el SUBVI llamado guardar datos de amplitud y tiempo."
                              n527 = Transpose 2D Array(2D array=w988) -> (transposed array=w990:string[][])
                              n528 = call <vilib>:"Three Button Dialog.vi"("Right Button Text (\"Cancel\")"="Señal EMG, potencia optica y distancia" ("Right Button Text (\"Cancel\")"), "Center Button Text (\"No\")"="Potencia optica y distancia" ("Center Button Text (\"No\")"), "Left Button Text (\"Yes\")"="Señal EMG" ("Left Button Text (\"Yes\")"), "message"="Elija que datos desea guardar") -> ("Which Button?"=w995:T3)  [unwired: 7 in]
                              n529 = case shown="\"Center Button\"" w995 {
                                tunnel: w994 -> [w1004 w1009 w1012]
                                tunnel: w993 -> [w1003 w1008 w1013]
                                tunnel: w992 -> [w1002 w1007 w1014]
                                tunnel: w991 -> [w1001 _ _]
                                tunnel: w990 -> [_ w1006 _]
                                tunnel: w989 -> [_ _ w1010]
                                frame "Left Button", Default {
                                # "Se guarda solo la señal EMG y su tiempo de adquisición."
                                n530 = call "Guardar datos de Amplitud y Tiempo.vi"("path"=w1004, "Hora inicio"=w1003, "Hora fin"=w1002, "Datos experimento"=w1001, "column headers"=string[] ["Tiempo(s)", "Amplitud(V)"]) -> ()  [unwired: 1 in]
                                }
                                frame "Center Button" {
                                # "Se guarda la potenica del lente derecho, del lente izquierdo, la distancia y el tiempo de estas variables."
                                n531 = call "Guardar datos de Amplitud y Tiempo.vi"("path"=w1009, "Hora inicio"=w1008, "Hora fin"=w1007, "Datos experimento"=w1006, "column headers"=string[] ["Tiempo(s)", "Distancia (cm)", "Potencia Optica derecho", "Potencia optica izquierdo"]) -> ()  [unwired: 1 in]
                                }
                                frame "Right Button" {
                                # "Se guarda el tiempo de adquisición así como la amplitud de la señal EMG,  la potenica del lente derecho, del lente izquierdo, la distancia y el tiempo de estas variables."
                                n532 = call "Guardar datos de Amplitud y Tiempo.vi"("path"=w1012, "Hora inicio"=w1013, "Hora fin"=w1014, "Datos experimento"=w1010, "column headers"=string[] ["Tiempo EMG(s)", "Amplitud(V)", "Tiempo DPT(s)", "Distancia (cm)", "Potencia optica derecho", "Potencia optica izquierdo"]) -> ()  [unwired: 1 in]
                                }
                              }
                            }
                            frame #2 {
                              # "Si el usuario desea repetir el experimento se vuelve al estado inicio en donde se espera que comience el experimento. De lo contrario se sale del loop y vuelve al menu principal."
                              n533 = Two Button Dialog(message="¿Desea repetir el experimento?", 1:"No" ("F button name (\"Cancel\")"), 2:"Si" ("T button name (\"OK\")")) -> (T button?=w1017:bool)
                              n534 = Not(x=w1017) -> (.not. x?=→"T button?":bool)
                            }
                          }
                        }
                      }
                      n535 = local read "T button?"() -> (w581:bool)
                    }
                  }
                }
                "Array 2" <- w483
              }
            }
          }
          event Timeout {
            n536 = event-data() -> ()  [unwired: 1 in, 3 out]
          }
        }
        "Array 3" <- w31
      }
      "Array 4" <- w22
    }
  }
